vi "Main[Top VI].vi"() -> ()   [LabVIEW 2011]
uses:
  <vilib>/picture/picture.llb/imagedata.ctl
  VIs/sub-Language global.vi
panel:
  out "selected":i32
  out "label4":string="统计数据：通道2"
  out "label3":string="统计数据：通道1"
  out "label2":string="CAN中继状态"
  out "label1":string="CAN发送"
  out "brgsta":u16(ring) caption="CAN中继状态"
  out "Trate2":dbl caption="帧率T:" format="%#.1f"
  out "Rrate2":dbl caption="帧率R:" format="%#.1f"
  out "errcnt2":i32 caption="校验错误:"
  out "Trate1":dbl caption="帧率T:" format="%#.1f"
  in  "path":path
  out "Rrate1":dbl caption="帧率R:" format="%#.1f"
  out "errcnt1":i32 caption="校验错误:"
  in  "reciveEnable":bool=TRUE
  in  "ID Filter Set":bool
  in  "ID Filter Str":string="01 02"
  in  "ID Filter":enum32{"enable", "disable"}(radio)=enum."disable" caption="接收滤波ID设置(直接ID号)"
  in  "savefile":bool
  in  "sendfile":bool
  in  "clear":bool
  in  "send stop":bool
  out "SaveCnt":u32 caption="保存总帧数:"
  in  "Send":bool
  in  "Data Inc":bool
  in  "sendcycle":i32=10 caption="发送周期:" min=0 max=99999999 step=1
  in  "data":string="00 00 00 00 00 00 00 00" caption="数据:"
  in  "ID Inc":bool
  in  "SendCnt":i32=1 caption="发送总帧数:" min=-1
  in  "CAN Channel":u16(ring) caption="CAN通道:" items=["1", "2"]
  in  "Frame ID":string="00 00 00 01" caption="帧ID:"
  in  "Frame Type":u16(ring) caption="帧类型:" items=["数据帧", "远程帧"]
  in  "Frame Format":u16(ring) caption="帧格式:" items=["标准帧", "扩展帧"]
  out "DevIndex":u32
  in  "list":i32(listbox)
  # "ms"
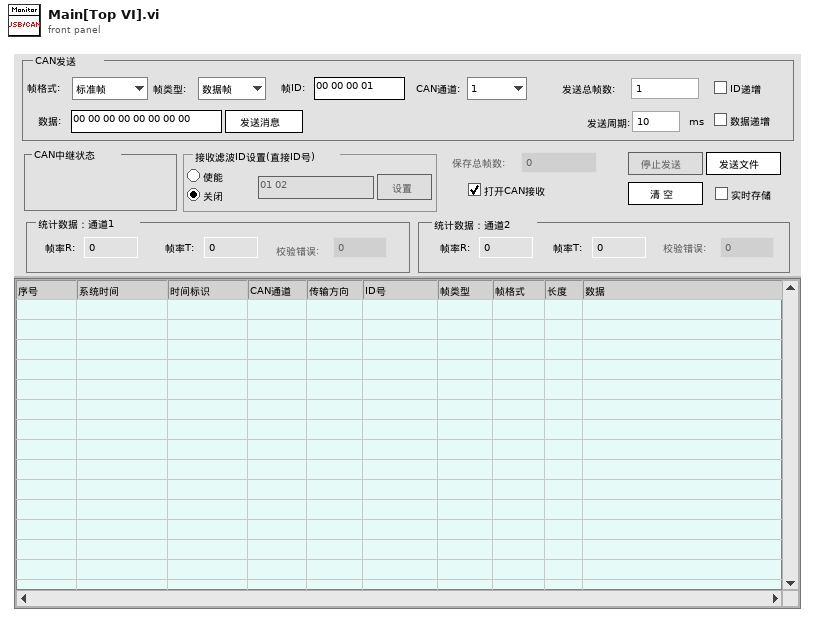
[diagram p1: front panel]
types:
  T1 = enum16{"Init", "RegistEvent", "run", "unRegistEvent", "Release", "Exit"}
  T2 = cluster{"type":u16, "scantime":u16, "highspd":bool, "disp":bool, "save":bool, "hl":bool, "ID合并":bool, "Rfun":u16, "Tfun":u16, "chk1":bool, "chk2":bool, "format":enum16{"hex", "dec", "oct", "bin"}, "rateR1":bool, "rateR2":bool, "rateT1":bool, "rateT2":bool, "RcvE1":bool, "RcvE2":bool, "TSFormat":enum16{"原始值", "实际值"}, "RcvLen":i16, "autoconn":bool, "BuffLen":u16}
  T3 = typedef "imagedata.ctl" = cluster{"image type":i32, "image depth":i32, "image":u8[], "mask":u8[], "colors":u32[], "Rectangle":cluster{"left":i16, "top":i16, "right":i16, "bottom":i16}}
  T4 = enum8{"Enabled", "Disabled", "Disabled and Grayed Out"}
  T5 = typedef "Param.ctl" = cluster{"kCANBAUD":u8, "BTR0":u8, "BTR1":u8, "MODE":u8, "FILTER":u8, "ACR0":u32, "AMR0":u32, "FlashParam":u32, "BAUD":u32, "SJW":u8, "BRP":u8, "SAM":u8, "PHS2_SEL":u8, "PRSEG":u8, "PHSEG1":u8, "PHSEG2":u8}
  T6 = cluster{"desc":string, "appended path":path, "help dir":string}[]
  T7 = cluster{"hw_Version":u16, "fw_Version":u16, "dr_Version":u16, "in_Version":u16, "irq_Num":u16, "can_Num":u8, "str_Serial_Num":string, "str_hw_Type":string, "Reserved":u8[]}
  T8 = cluster{"desc":string, "appended path":path, "help dir":string}
  T9 = enum16{"X", "CAN1--->CAN2", "CAN1<----CAN2", "CAN1<---->CAN2"}
  T10 = typedef "LVPoint32TypeDef.ctl" = cluster{"Horizontal":i32, "Vertical":i32}
  T11 = typedef "LVRowAndColumnTypeDef.ctl" = cluster{"Row":i32, "Column":i32}
  T12 = enum32{"Bad", "Idle", "Run top level", "Running"}
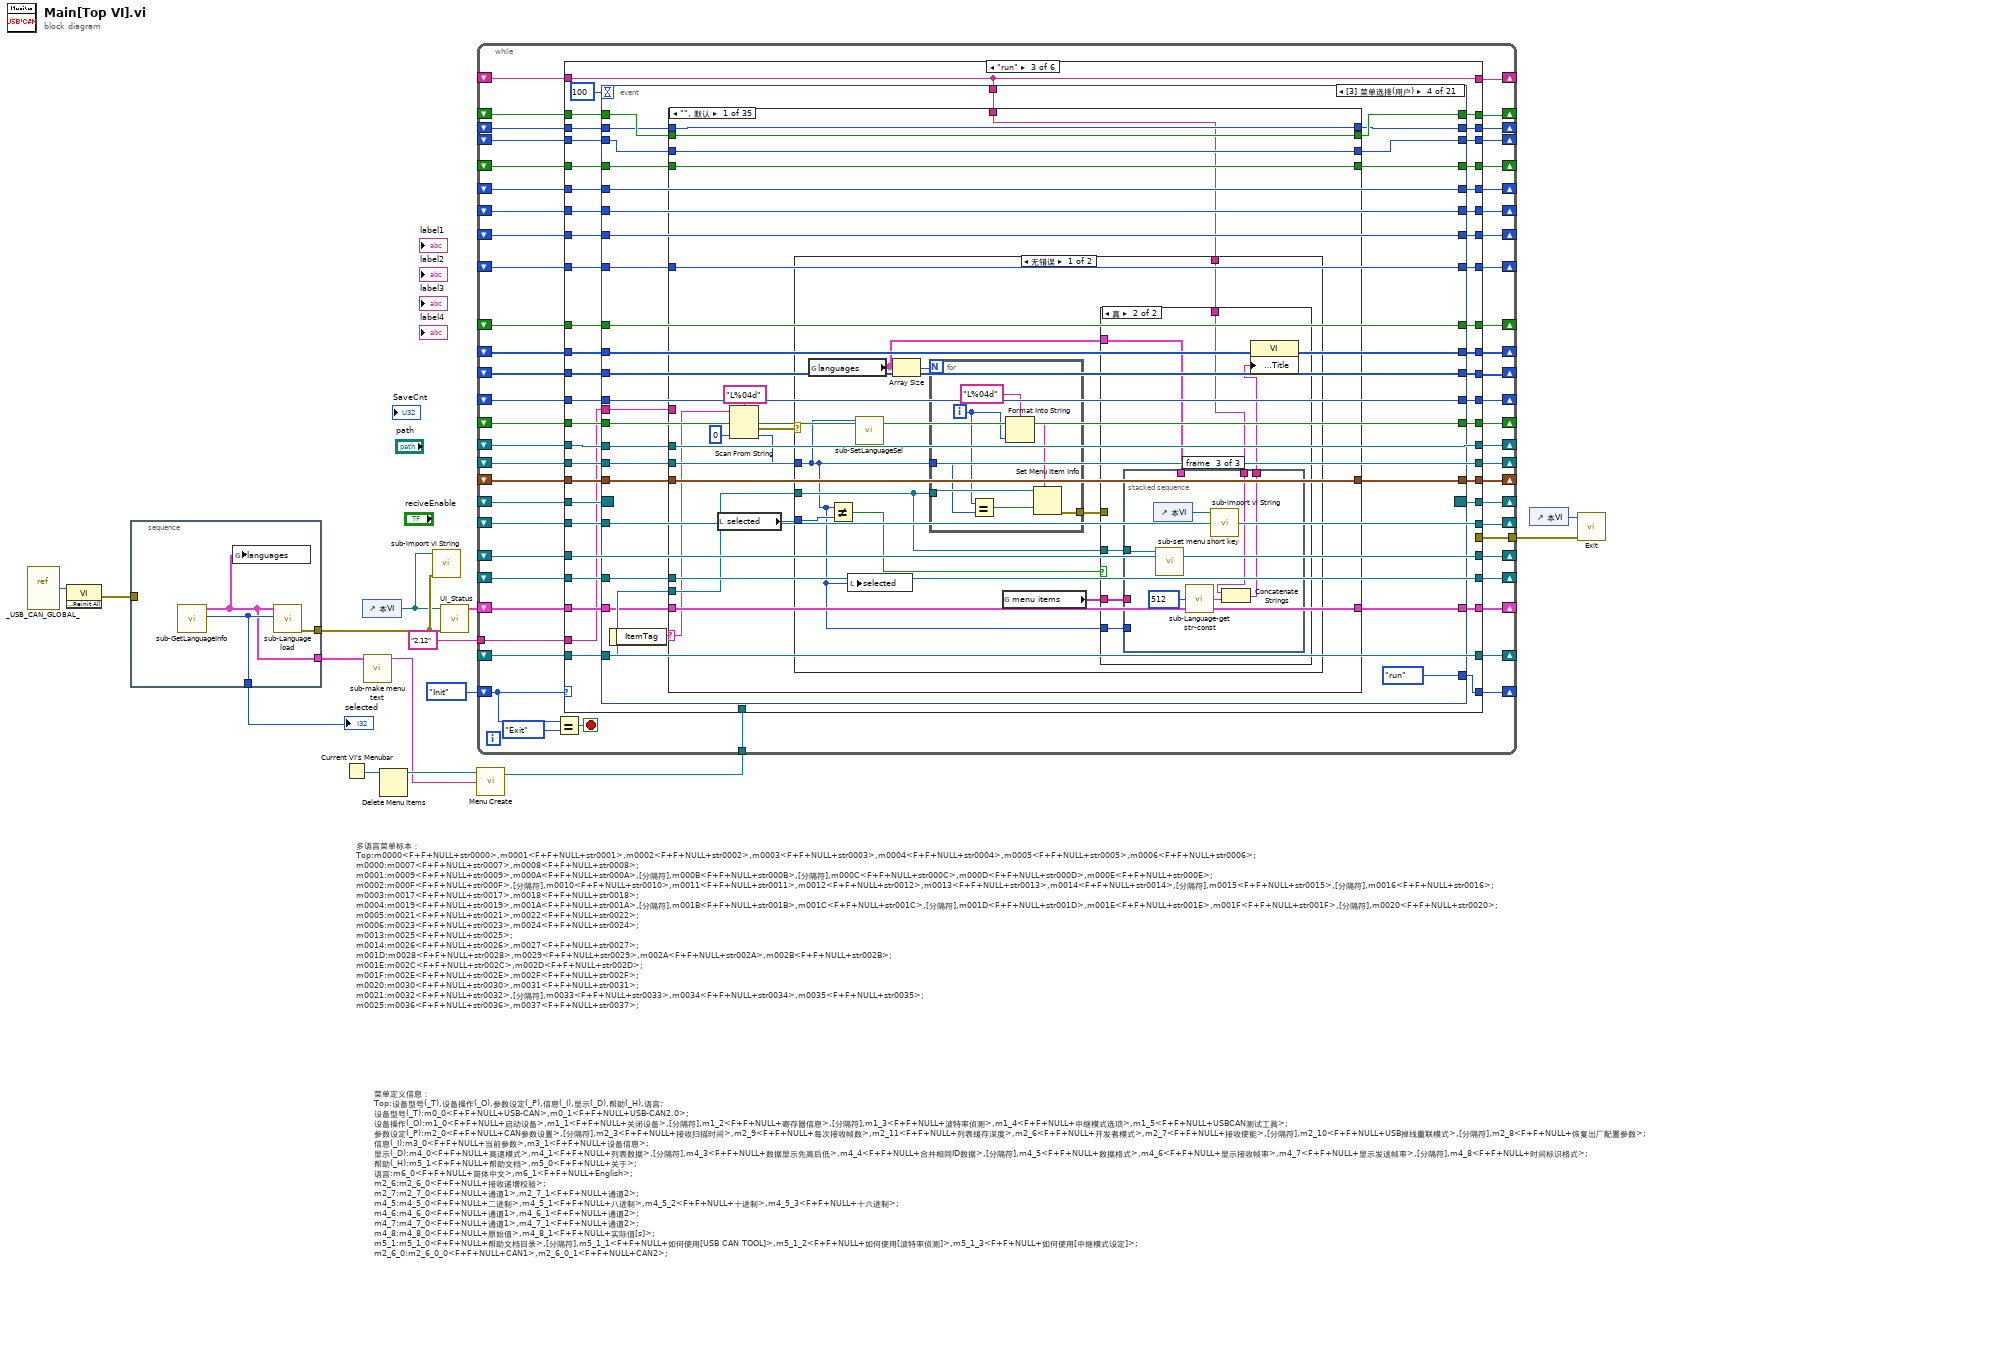
[diagram p0: block diagram]
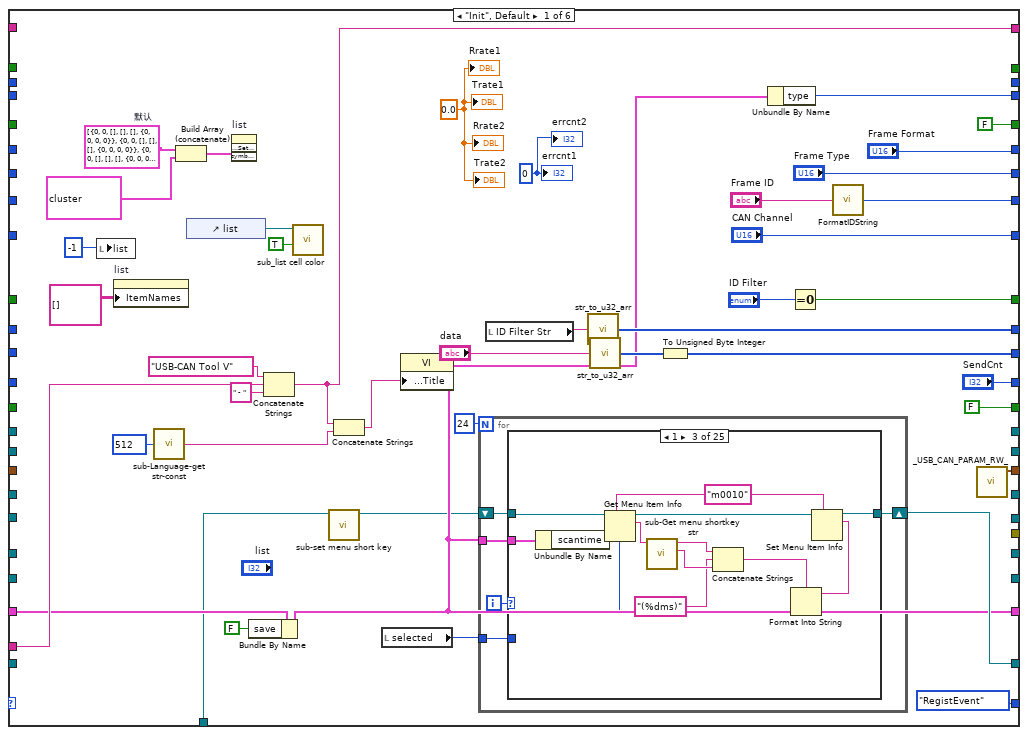
[diagram p2: hidden frame]
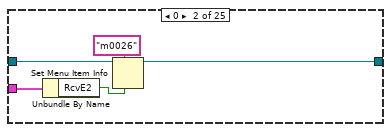
[diagram p4: hidden frame]
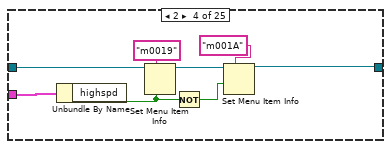
[diagram p5: hidden frame]
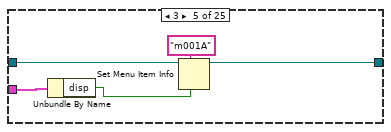
[diagram p6: hidden frame]
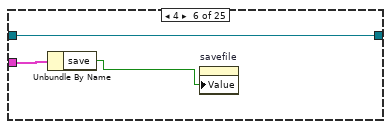
[diagram p7: hidden frame]
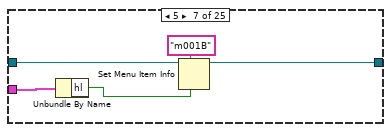
[diagram p8: hidden frame]
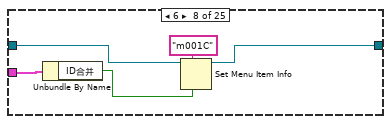
[diagram p9: hidden frame]
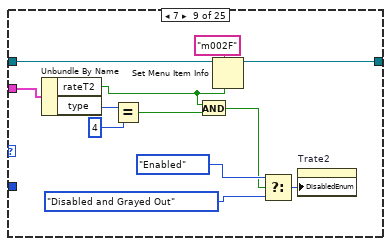
[diagram p10: hidden frame]
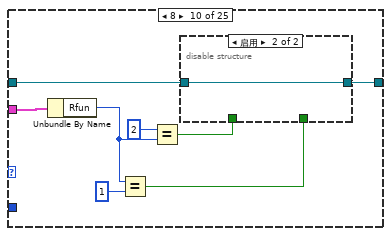
[diagram p11: hidden frame]
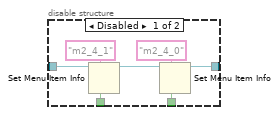
[diagram p12: hidden frame]
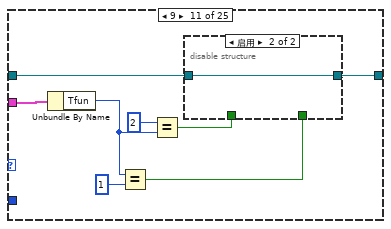
[diagram p13: hidden frame]
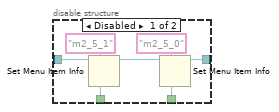
[diagram p14: hidden frame]
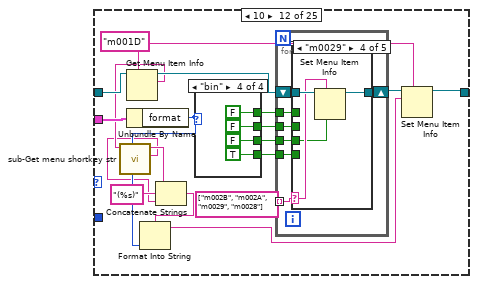
[diagram p15: hidden frame]
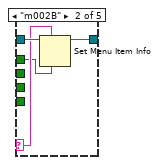
[diagram p17: hidden frame]
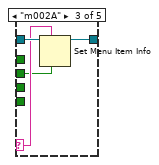
[diagram p18: hidden frame]
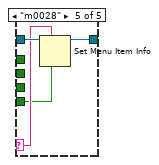
[diagram p19: hidden frame]
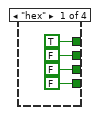
[diagram p20: hidden frame]
diagram:
  # "菜单定义信息：\nTop:设备型号(_T),设备操作(_O),参数设定(_P),信息(_I),显示(_D),帮助(_H),语言;\n设备型号(_T):m0_0<F+F+NULL+USB-CAN>,m0_1<F+F+NULL+USB-CAN2.0>;\n设备操作(_O):m1_0<F+F+NULL+启动设备>,m1_1<F+F+NULL+关闭设备>,[分隔符],m1_2<F+F+NULL+寄存器信息>,[分隔符],m1_3<F+F+NULL+波特率侦测>,m1_4<F+F+NULL+中继模式选项>,m1_5<F+F+NULL+USBCAN测试工具>;\n参数设定(_P):m2_0<F+F+NULL+CAN参数设置>,[分隔符],m2_3<F+F+NULL+接收扫描时间>,m2_9<F+F+NULL+每次接收帧数>,m2_11<F+F+NULL+列表缓存深度>,m2_6<F+F+NULL+开发者模式>,m2_7<F+F+NULL+接收使能>,[分隔符],m2_10<F+F+NULL+USB掉线重联模式>,[分隔符],m2_8<F+F+NULL+恢复出厂配置参数>;\n信息(_I):m3_0<F+F+NULL+当前参数>,m3_1<F+F+NULL+设备信息>;\n显示(_D):m4_0<F+F+NULL+高速模式>,m4_1<F+F+NULL+列表数据>,[分隔符],m4_3<F+F+NULL+数据显示先高后低>,m4_4<F+F+NULL+合并相同ID数据>,[分隔符],m4_5<F+F+NULL+数据格式>,m4_6<F+F+NULL+显示接收帧率>,m4_7<F+F+NULL+显示发送帧率>,[分隔符],m4_8<F+F+NULL+时间标识格式>;\n帮助(_H):m5_1<F+F+NULL+帮助文档>,m5_0<F+F+NULL+关于>;\n语言:m6_0<F+F+NULL+简体中文>,m6_1<F+F+NULL+English>;\nm2_6:m2_6_0<F+F+NULL+接收递增校验>;\nm2_7:m2_7_0<F+F+NULL+通道1>,m2_7_1<F+F+NULL+通道2>;\nm4_5:m4_5_0<F+F+NULL+二进制>,m4_5_1<F+F+NULL+八进制>,m4_5_2<F+F+NULL+十进制>,m4_5_3<F+F+NULL+十六进制>;\nm4_6:m4_6_0<F+F+NULL+通道1>,m4_6_1<F+F+NULL+通道2>;\nm4_7:m4_7_0<F+F+NULL+通道1>,m4_7_1<F+F+NULL+通道2>;\nm4_8:m4_8_0<F+F+NULL+原始值>,m4_8_1<F+F+NULL+实际值[s]>;\nm5_1:m5_1_0<F+F+NULL+帮助文档目录>,[分隔符],m5_1_1<F+F+NULL+如何使用[USB CAN TOOL]>,m5_1_2<F+F+NULL+如何使用[波特率侦测]>,m5_1_3<F+F+NULL+如何使用[中继模式设定]>;\nm2_6_0:m2_6_0_0<F+F+NULL+CAN1>,m2_6_0_1<F+F+NULL+CAN2>;"
  # "多语言菜单标本：\nTop:m0000<F+F+NULL+str0000>,m0001<F+F+NULL+str0001>,m0002<F+F+NULL+str0002>,m0003<F+F+NULL+str0003>,m0004<F+F+NULL+str0004>,m0005<F+F+NULL+str0005>,m0006<F+F+NULL+str0006>;\nm0000:m0007<F+F+NULL+str0007>,m0008<F+F+NULL+str0008>;\nm0001:m0009<F+F+NULL+str0009>,m000A<F+F+NULL+str000A>,[分隔符],m000B<F+F+NULL+str000B>,[分隔符],m000C<F+F+NULL+str000C>,m000D<F+F+NULL+str000D>,m000E<F+F+NULL+str000E>;\nm0002:m000F<F+F+NULL+str000F>,[分隔符],m0010<F+F+NULL+str0010>,m0011<F+F+NULL+str0011>,m0012<F+F+NULL+str0012>,m0013<F+F+NULL+str0013>,m0014<F+F+NULL+str0014>,[分隔符],m0015<F+F+NULL+str0015>,[分隔符],m0016<F+F+NULL+str0016>;\nm0003:m0017<F+F+NULL+str0017>,m0018<F+F+NULL+str0018>;\nm0004:m0019<F+F+NULL+str0019>,m001A<F+F+NULL+str001A>,[分隔符],m001B<F+F+NULL+str001B>,m001C<F+F+NULL+str001C>,[分隔符],m001D<F+F+NULL+str001D>,m001E<F+F+NULL+str001E>,m001F<F+F+NULL+str001F>,[分隔符],m0020<F+F+NULL+str0020>;\nm0005:m0021<F+F+NULL+str0021>,m0022<F+F+NULL+str0022>;\nm0006:m0023<F+F+NULL+str0023>,m0024<F+F+NULL+str0024>;\nm0013:m0025<F+F+NULL+str0025>;\nm0014:m0026<F+F+NULL+str0026>,m0027<F+F+NULL+str0027>;\nm001D:m0028<F+F+NULL+str0028>,m0029<F+F+NULL+str0029>,m002A<F+F+NULL+str002A>,m002B<F+F+NULL+str002B>;\nm001E:m002C<F+F+NULL+str002C>,m002D<F+F+NULL+str002D>;\nm001F:m002E<F+F+NULL+str002E>,m002F<F+F+NULL+str002F>;\nm0020:m0030<F+F+NULL+str0030>,m0031<F+F+NULL+str0031>;\nm0021:m0032<F+F+NULL+str0032>,[分隔符],m0033<F+F+NULL+str0033>,m0034<F+F+NULL+str0034>,m0035<F+F+NULL+str0035>;\nm0025:m0036<F+F+NULL+str0036>,m0037<F+F+NULL+str0037>;"
  n1 = vi-ref "_USB_CAN_GLOBAL_.vi"() -> (w7:refnum<vi>)
  n2 = invoke class="VI" method="Default Vals.Reinit All"(reference=w7) -> (error out=w5:errorcluster)  [unwired: 2 in, 2 out]
  n3 = stacked-sequence {
    tunnel: [w18] -> w10
    tunnel: [w17] -> w8
    tunnel: [w16] -> w6
    tunnel: w5 -> [_]
    frame #0 {
      n4 = call "sub-GetLanguageInfo.vi"() -> ("selected"=w17:i32, "languages"=w16:cluster{string, "appended path":path, string}[])  [unwired: 10 in]
      n5 = global write "sub-Language global.vi" "languages"(w16) -> ()
      n6 = call "sub-Language load.vi"("selected"=w17, "languages"=w16) -> ("error out"=w18:errorcluster)  [unwired: 9 in]
    }
  }
  "selected" <- w8
  n7 = Current VI's Menubar() -> (w4:refnum<k9>)
  n8 = control-ref of="本VI"() -> (w9:refnum<vi>)
  n9 = call "sub-make menu text.vi"("languages"=w6) -> ("menu text"=w2:string)  [unwired: 10 in]
  n10 = Delete Menu Items(9:w4) -> (3:w3:refnum<k9>)  [unwired: 1 in, 3 out]
  n11 = call "sub-import vi String.vi"("error in (no error)"=w10, "vi ref"=w9) -> ()  [unwired: 9 in, 1 out]
  n12 = call "UI_Status.vi"("error in (no error)"=w10, "VI ref"=w9) -> ("menu status in out"=w14:T2)  [unwired: 8 in, 1 out]
  n13 = call "Menu Create.vi"("String"=w2, "menubar in"=w3) -> ("menubar out"=w1:refnum<k9>)  [unwired: 1 in, 1 out]
  n14 = while {
    shift-right: [w68] -> _
    shift-left: T1."Init" -> [w71]
    shift-right: [w67] -> _
    shift-left: _ -> [w66]
    shift-right: [w64] -> _
    shift-left: _ -> [w65]
    shift-right: [w63] -> _
    shift-left: _ -> [w62]
    shift-right: [w61] -> _
    shift-left: _ -> [w60]
    shift-right: [w59] -> _
    shift-left: _ -> [w58]
    shift-right: [w57] -> _
    shift-left: _ -> [w56]
    shift-right: [w55] -> _
    shift-left: _ -> [w54]
    shift-right: [w53] -> _
    shift-left: _ -> [w52]
    shift-right: [w51] -> _
    shift-left: _ -> [w50]
    shift-right: [w49] -> _
    shift-left: _ -> [w48]
    shift-right: [w47] -> _
    shift-left: _ -> [w46]
    shift-right: [w44] -> _
    shift-left: _ -> [w45]
    shift-right: [w43] -> _
    shift-left: _ -> [w42]
    shift-right: [w41] -> _
    shift-left: _ -> [w40]
    shift-right: [w39] -> _
    shift-left: _ -> [w38]
    shift-right: [w37] -> _
    shift-left: _ -> [w35]
    shift-right: [w36] -> _
    shift-left: _ -> [w34]
    tunnel: [w33] -> w13
    shift-right: [w32] -> _
    shift-left: _ -> [w31]
    shift-right: [w30] -> _
    shift-left: w14 -> [w29]
    shift-right: [w28] -> _
    shift-left: _ -> [w27]
    shift-right: [w26] -> _
    shift-left: _ -> [w25]
    shift-right: [w24] -> _
    shift-left: _ -> [w23]
    shift-right: [w22] -> _
    shift-left: _ -> [w21]
    tunnel: "2.12" ("FileVersion") -> [w20]
    tunnel: w1 -> [w19]
    stop <- w69 stop-if-true
    n15 = Equal?(x=w71, y=T1."Exit") -> (x = y?=w69:bool)
    n16 = case shown="\"run\"" w71 {
      tunnel: [T1."RegistEvent" T1."run" w767 T1."Release" T1."Exit" T1."Exit"] -> w68
      tunnel: [FALSE w468 w776 _ _ _] -> w67
      tunnel: w66 -> [_ w468 w785 _ _ _]
      tunnel: w65 -> [_ w467 w784 _ _ _]
      tunnel: ["Frame Format" w467 w775 _ _ _] -> w64
      tunnel: ["Frame Type" w455 w774 _ _ _] -> w63
      tunnel: w62 -> [_ w455 w783 _ _ _]
      tunnel: [w108 w466 w773 _ _ _] -> w61
      tunnel: w60 -> [_ w466 w782 _ _ _]
      tunnel: ["CAN Channel" w454 w772 _ _ _] -> w59
      tunnel: w58 -> [_ w454 w781 _ _ _]
      tunnel: [w84 w441 w770 _ _ _] -> w57
      tunnel: w56 -> [_ w441 w779 _ _ _]
      tunnel: [w105 w442 w771 _ _ _] -> w55
      tunnel: w54 -> [_ w442 w780 _ _ _]
      tunnel: [w99 w465 w769 _ _ _] -> w53
      tunnel: w52 -> [_ w465 w778 _ _ _]
      tunnel: ["SendCnt" w464 w768 _ _ _] -> w51
      tunnel: w50 -> [_ w464 w777 _ _ _]
      tunnel: [FALSE w463 w765 _ _ _] -> w49
      tunnel: w48 -> [_ w463 w766 _ _ _]
      tunnel: [w91 w462 w752 w2340 w2388 _] -> w47
      tunnel: w46 -> [_ w462 w752 w2340 w2388 _]
      tunnel: w45 -> [_ w461 w764 w2334 _ _]
      tunnel: [w86 w461 w763 _ _ _] -> w44
      tunnel: [_ w445 w762 _ _ _] -> w43
      tunnel: w42 -> [_ _ w762 w2358 _ _]
      tunnel: [_ w444 w761 _ _ _] -> w41
      tunnel: w40 -> [_ _ w761 w2351 _ _]
      tunnel: [w96 w456 w759 _ _ _] -> w39
      tunnel: w38 -> [_ w456 w760 w2342 _ _]
      tunnel: [_ w452 w757 _ _ _] -> w37
      tunnel: [_ w451 w756 _ _ _] -> w36
      tunnel: w35 -> [_ _ w758 w2348 _ _]
      tunnel: w34 -> [_ _ w756 w2346 _ _]
      tunnel: [_ _ _ w2345 _ _] -> w33
      tunnel: [_ w446 w755 _ _ _] -> w32
      tunnel: w31 -> [_ _ w755 w2343 _ _]
      tunnel: [w83 w421 w753 w2339 _ _] -> w30
      tunnel: w29 -> [w85 w421 w754 w2339 w2385 _]
      tunnel: [_ FALSE w750 _ _ _] -> w28
      tunnel: w27 -> [_ _ w751 _ _ _]
      tunnel: [_ w433 w749 _ _ _] -> w26
      tunnel: w25 -> [_ _ w749 w2337 _ _]
      tunnel: [_ _ w747 _ _ _] -> w24
      tunnel: w23 -> [_ _ w748 _ _ _]
      tunnel: [w74 w413 w746 w2336 w2384 w2394] -> w22
      tunnel: w21 -> [_ w413 w746 w2336 w2384 w2394]
      tunnel: w20 -> [w89 _ w745 _ _ _]
      tunnel: w19 -> [w77 _ _ _ _ _]
      frame "Init", Default {
        w87 = 0.0 ("rate")
        w95 = T3[] [{"image type"=0, "image depth"=0, "image"=[], "mask"=[], "colors"=[], "Rectangle"={"left"=0, "top"=0, "right"=0, "bottom"=0}}, {"image type"=0, "image depth"=0, "image"=[], "mask"=[], "colors"=[], "Rectangle"={"left"=0, "top"=0, "right"=0, "bottom"=0}}, {"image type"=0, "image depth"=0, "image"=[], "mask"=[], "colors"=[], "Rectangle"={"left"=0, "top"=0, "right"=0, "bottom"=0}}, {"image type"=0, "image depth"=0, "image"=[], "mask"=[], "colors"=[], "Rectangle"={"left"=0, "top"=0, "right"=0, "bottom"=0}}, {"image type"=0, "image depth"=0, "image"=[], "mask"=[], "colors"=[], "Rectangle"={"left"=0, "top"=0, "right"=0, "bottom"=0}}, {"image type"=0, "image depth"=0, "image"=[], "mask"=[], "colors"=[], "Rectangle"={"left"=0, "top"=0, "right"=0, "bottom"=0}}, {"image type"=0, "image depth"=0, "image"=[], "mask"=[], "colors"=[], "Rectangle"={"left"=0, "top"=0, "right"=0, "bottom"=0}}, {"image type"=0, "image depth"=0, "image"=[], "mask"=[], "colors"=[], "Rectangle"={"left"=0, "top"=0, "right"=0, "bottom"=0}}, {"image type"=0, "image depth"=0, "image"=[], "mask"=[], "colors"=[], "Rectangle"={"left"=0, "top"=0, "right"=0, "bottom"=0}}, {"image type"=0, "image depth"=0, "image"=[], "mask"=[], "colors"=[], "Rectangle"={"left"=0, "top"=0, "right"=0, "bottom"=0}}, {"image type"=0, "image depth"=0, "image"=[], "mask"=[], "colors"=[], "Rectangle"={"left"=0, "top"=0, "right"=0, "bottom"=0}}, {"image type"=0, "image depth"=0, "image"=[], "mask"=[], "colors"=[], "Rectangle"={"left"=0, "top"=0, "right"=0, "bottom"=0}}, {"image type"=0, "image depth"=0, "image"=[], "mask"=[], "colors"=[], "Rectangle"={"left"=0, "top"=0, "right"=0, "bottom"=0}}, {"image type"=0, "image depth"=0, "image"=[], "mask"=[], "colors"=[], "Rectangle"={"left"=0, "top"=0, "right"=0, "bottom"=0}}, {"image type"=0, "image depth"=0, "image"=[], "mask"=[], "colors"=[], "Rectangle"={"left"=0, "top"=0, "right"=0, "bottom"=0}}, {"image type"=0, "image depth"=0, "image"=[], "mask"=[], "colors"=[], "Rectangle"={"left"=0, "top"=0, "right"=0, "bottom"=0}}, {"image type"=0, "image depth"=0, "image"=[], "mask"=[], "colors"=[], "Rectangle"={"left"=0, "top"=0, "right"=0, "bottom"=0}}, {"image type"=0, "image depth"=0, "image"=[], "mask"=[], "colors"=[], "Rectangle"={"left"=0, "top"=0, "right"=0, "bottom"=0}}, {"image type"=0, "image depth"=0, "image"=[], "mask"=[], "colors"=[], "Rectangle"={"left"=0, "top"=0, "right"=0, "bottom"=0}}, {"image type"=0, "image depth"=0, "image"=[], "mask"=[], "colors"=[], "Rectangle"={"left"=0, "top"=0, "right"=0, "bottom"=0}}, {"image type"=0, "image depth"=0, "image"=[], "mask"=[], "colors"=[], "Rectangle"={"left"=0, "top"=0, "right"=0, "bottom"=0}}, {"image type"=0, "image depth"=0, "image"=[], "mask"=[], "colors"=[], "Rectangle"={"left"=0, "top"=0, "right"=0, "bottom"=0}}, {"image type"=0, "image depth"=0, "image"=[], "mask"=[], "colors"=[], "Rectangle"={"left"=0, "top"=0, "right"=0, "bottom"=0}}, {"image type"=0, "image depth"=0, "image"=[], "mask"=[], "colors"=[], "Rectangle"={"left"=0, "top"=0, "right"=0, "bottom"=0}}, {"image type"=0, "image depth"=0, "image"=[], "mask"=[], "colors"=[], "Rectangle"={"left"=0, "top"=0, "right"=0, "bottom"=0}}, {"image type"=0, "image depth"=0, "image"=[], "mask"=[], "colors"=[], "Rectangle"={"left"=0, "top"=0, "right"=0, "bottom"=0}}, {"image type"=0, "image depth"=0, "image"=[], "mask"=[], "colors"=[], "Rectangle"={"left"=0, "top"=0, "right"=0, "bottom"=0}}, {"image type"=0, "image depth"=0, "image"=[], "mask"=[], "colors"=[], "Rectangle"={"left"=0, "top"=0, "right"=0, "bottom"=0}}, {"image type"=0, "image depth"=0, "image"=[], "mask"=[], "colors"=[], "Rectangle"={"left"=0, "top"=0, "right"=0, "bottom"=0}}, {"image type"=0, "image depth"=0, "image"=[], "mask"=[], "colors"=[], "Rectangle"={"left"=0, "top"=0, "right"=0, "bottom"=0}}, {"image type"=0, "image depth"=0, "image"=[], "mask"=[], "colors"=[], "Rectangle"={"left"=0, "top"=0, "right"=0, "bottom"=0}}, {"image type"=0, "image depth"=0, "image"=[], "mask"=[], "colors"=[], "Rectangle"={"left"=0, "top"=0, "right"=0, "bottom"=0}}, {"image type"=0, "image depth"=0, "image"=[], "mask"=[], "colors"=[], "Rectangle"={"left"=0, "top"=0, "right"=0, "bottom"=0}}, {"image type"=0, "image depth"=0, "image"=[], "mask"=[], "colors"=[], "Rectangle"={"left"=0, "top"=0, "right"=0, "bottom"=0}}, {"image type"=0, "image depth"=0, "image"=[], "mask"=[], "colors"=[], "Rectangle"={"left"=0, "top"=0, "right"=0, "bottom"=0}}, {"image type"=0, "image depth"=0, "image"=[], "mask"=[], "colors"=[], "Rectangle"={"left"=0, "top"=0, "right"=0, "bottom"=0}}, {"image type"=0, "image depth"=0, "image"=[], "mask"=[], "colors"=[], "Rectangle"={"left"=0, "top"=0, "right"=0, "bottom"=0}}]  # 默认
        w88 = 0 ("errcnt")
        n17 = local write "list"(-1 ("list")) -> ()
        n18 = property on="list" class="MCListbox (严格)"("ItemNames"=string[][] [] ("项名")) -> ()  [unwired: 2 in, 2 out]
        n19 = call "sub-Language-get str-const.vi"("sid"=u32 512) -> ("str"=w73:string)
        n20 = Build Array (concatenate)(w95, T3[] [{"image type"=0, "image depth"=32, "image"=array[1024 elements], "mask"=[255, 255, 255, 255, 255, 255, 255, 255, 255, 255, 255, 255, 255, 255, 255, 255, 255, 255, 255, 255, 255, 255, 255, 255, 255, 255, 255, 255, 255, 255, 255, 255], "colors"=[], "Rectangle"={"left"=0, "top"=0, "right"=16, "bottom"=16}}, {"image type"=0, "image depth"=32, "image"=array[1024 elements], "mask"=[255, 255, 255, 255, 255, 255, 255, 255, 255, 255, 255, 255, 255, 255, 255, 255, 255, 255, 255, 255, 255, 255, 255, 255, 255, 255, 255, 255, 255, 255, 255, 255], "colors"=[], "Rectangle"={"left"=0, "top"=0, "right"=16, "bottom"=16}}] ("数组")) -> (w94:T3[])
        n21 = control-ref of="list"() -> (w81:refnum<vi>)
        n22 = invoke on="list" class="MCListbox (严格)" method="Custom Item Symbols.Set Symbol Array"("symbols"=w94) -> ()  [unwired: 3 in, 4 out]
        n23 = Bundle By Name(cluster=w85, "save"=FALSE) -> (w83:T2)
        n24 = Concatenate Strings("USB-CAN Tool V", w89, " - " ("字符串")) -> (w74:string)
        n25 = call "sub_list cell color.vi"("Reset?(F)"=TRUE, "list ref"=w81) -> ()  [unwired: 8 in, 2 out]
        n26 = call "sub-set menu short key.vi"("menubar in"=w77) -> ("menubar out"=w78:refnum<k9>)  [unwired: 9 in, 1 out]
        n27 = Concatenate Strings(w74, w73) -> (w72:string)
        n28 = local read "selected"() -> (w79:i32)
        n29 = property class="VI"("Front Panel.Title"=w72) -> ()  [unwired: 2 in, 2 out]
        n30 = for {
          N: 24 -> [_]
          shift-right: [w115] -> w91
          shift-left: w78 -> [w116]
          tunnel: w83 -> [w117]
          tunnel: w79 -> [w114]
          i -> [w118]
          n31 = case shown="1" w118 {
            tunnel: w117 -> [_ w124 w136 w144 w149 w152 w157 w162 w174 w182 w198 w224 w272 w284 w292 w304 w312 w317 w334 _ w370 w387 w399 w402 _]
            tunnel: w116 -> [w119 w123 w132 w143 w148 w151 w156 w161 w173 w181 w197 w214 w271 w283 w291 w303 w311 w316 w332 w357 w376 w384 w396 w405 w411]
            tunnel: [w119 w121 w135 w140 w147 w151 w155 w160 w171 w180 w196 w217 w269 w281 w289 w301 w309 w314 w331 w356 w372 w388 w400 w404 w410] -> w115
            tunnel: w114 -> [_ _ _ _ _ _ _ _ _ _ _ _ _ _ _ _ _ _ _ _ _ _ _ _ w409]
            frame -1, Default {
            }
            frame 0 {
              n32 = Unbundle By Name(w124) -> ("RcvE2"=w120:bool)
              n33 = Set Menu Item Info(6:w120, 7:"m0026" ("项标识符"), 11:w123) -> (3:w121:refnum<k9>)  [unwired: 4 in, 1 out]
            }
            frame 1 {
              w130 = "m0010" ("项标识符")
              n34 = Unbundle By Name(w136) -> ("scantime"=w134:u16)
              n35 = Get Menu Item Info(7:w130, 11:w132) -> (2:w129:string, 3:w131:refnum<k9>)  [unwired: 1 in, 5 out]
              n36 = call "sub-Get menu shortkey str.vi"("menu desc"=w129) -> ("short key str"=w127:string, "menu desc split"=w128:string)  [unwired: 9 in]
              n37 = Concatenate Strings(w128, "(%dms)" ("格式字符串"), w127) -> (w125:string)
              n38 = Format Into String(format string=w125, w134) -> (resulting string=w133:string)  [unwired: 2 in, 1 out]
              n39 = Set Menu Item Info(7:w130, 10:w133, 11:w131) -> (3:w135:refnum<k9>)  [unwired: 4 in, 1 out]
            }
            frame 2 {
              n40 = Unbundle By Name(w144) -> ("highspd"=w138:bool)
              n41 = Set Menu Item Info(6:w138, 7:"m0019" ("项标识符"), 11:w143) -> (3:w141:refnum<k9>)  [unwired: 4 in, 1 out]
              n42 = Not(x=w138) -> (.not. x?=w137:bool)
              n43 = Set Menu Item Info(7:"m001A" ("项标识符"), 9:w137, 11:w141) -> (3:w140:refnum<k9>)  [unwired: 4 in, 1 out]
            }
            frame 3 {
              n44 = Unbundle By Name(w149) -> ("disp"=w145:bool)
              n45 = Set Menu Item Info(6:w145, 7:"m001A" ("项标识符"), 11:w148) -> (3:w147:refnum<k9>)  [unwired: 4 in, 1 out]
            }
            frame 4 {
              n46 = Unbundle By Name(w152) -> ("save"=w150:bool)
              n47 = property on="savefile" class="Bool (严格)"("Value"=w150) -> ()  [unwired: 2 in, 2 out]
            }
            frame 5 {
              n48 = Unbundle By Name(w157) -> ("hl"=w153:bool)
              n49 = Set Menu Item Info(6:w153, 7:"m001B" ("项标识符"), 11:w156) -> (3:w155:refnum<k9>)  [unwired: 4 in, 1 out]
            }
            frame 6 {
              n50 = Unbundle By Name(w162) -> ("ID合并"=w158:bool)
              n51 = Set Menu Item Info(6:w158, 7:"m001C" ("项标识符"), 11:w161) -> (3:w160:refnum<k9>)  [unwired: 4 in, 1 out]
            }
            frame 7 {
              n52 = Unbundle By Name(w174) -> ("rateT2"=w165:bool, "type"=w167:u16)
              n53 = Equal?(x=w167, y=u16 4) -> (x = y?=w164:bool)
              n54 = And(x=w165, y=w164) -> (x .and. y?=w163:bool)
              n55 = Set Menu Item Info(6:w165, 7:"m002F" ("项标识符"), 11:w173) -> (3:w171:refnum<k9>)  [unwired: 4 in, 1 out]
              n56 = Select(t=T4."Enabled" ("禁用"), s=w163, f=T4."Disabled and Grayed Out" ("禁用")) -> (s? t:f=w169:T4)
              n57 = property on="Trate2" class="DigNum (严格)"("DisabledEnum"=w169) -> ()  [unwired: 2 in, 2 out]
            }
            frame 8 {
              n58 = Unbundle By Name(w182) -> ("Rfun"=w177:u16)
              n59 = Equal?(x=w177, y=u16 1) -> (x = y?=w178:bool)
              n60 = Equal?(x=u16 2, y=w177) -> (x = y?=w175:bool)
              n61 = disable-structure shown="启用" {
                disable-tunnel: w181 -> [w189 w190]
                disable-tunnel: [w185 w190] -> w180
                disable-tunnel: w178 -> [w184 _]
                disable-tunnel: w175 -> [w183 _]
                frame Disabled {
                  n62 = Set Menu Item Info(6:w183, 7:"m2_4_1" ("项标识符"), 11:w189) -> (3:w186:refnum<k9>)  [unwired: 4 in, 1 out]
                  n63 = Set Menu Item Info(6:w184, 7:"m2_4_0" ("项标识符"), 11:w186) -> (3:w185:refnum<k9>)  [unwired: 4 in, 1 out]
                }
                frame Enabled {
                }
              }
            }
            frame 9 {
              n64 = Unbundle By Name(w198) -> ("Tfun"=w193:u16)
              n65 = Equal?(x=w193, y=u16 1) -> (x = y?=w194:bool)
              n66 = Equal?(x=u16 2, y=w193) -> (x = y?=w191:bool)
              n67 = disable-structure shown="启用" {
                disable-tunnel: w197 -> [w205 w206]
                disable-tunnel: [w201 w206] -> w196
                disable-tunnel: w194 -> [w200 _]
                disable-tunnel: w191 -> [w199 _]
                frame Disabled {
                  n68 = Set Menu Item Info(6:w199, 7:"m2_5_1" ("项标识符"), 11:w205) -> (3:w202:refnum<k9>)  [unwired: 4 in, 1 out]
                  n69 = Set Menu Item Info(6:w200, 7:"m2_5_0" ("项标识符"), 11:w202) -> (3:w201:refnum<k9>)  [unwired: 4 in, 1 out]
                }
                frame Enabled {
                }
              }
            }
            frame 10 {
              w212 = "m001D" ("项标识符")
              n70 = Get Menu Item Info(7:w212, 11:w214) -> (2:w211:string, 3:w213:refnum<k9>)  [unwired: 1 in, 5 out]
              n71 = call "sub-Get menu shortkey str.vi"("menu desc"=w211) -> ("short key str"=w208:string, "menu desc split"=w210:string)  [unwired: 9 in]
              n72 = Unbundle By Name(w224) -> ("format"=w219:enum16{"hex", "dec", "oct", "bin"})
              n73 = Concatenate Strings(w210, "(%s)" ("字符串"), w208) -> (w207:string)
              n74 = Format Into String(format string=w207, w219) -> (resulting string=w216:string)  [unwired: 2 in, 1 out]
              n75 = case shown="\"bin\"" w219 {
                tunnel: [TRUE FALSE FALSE FALSE] -> w223
                tunnel: [FALSE TRUE FALSE FALSE] -> w222
                tunnel: [FALSE FALSE TRUE FALSE] -> w221
                tunnel: [FALSE FALSE FALSE TRUE] -> w220
                frame "hex" {
                }
                frame "dec" {
                }
                frame "oct" {
                }
                frame "bin" {
                }
              }
              n76 = for {
                shift-right: [w230] -> w218
                shift-left: w213 -> [w231]
                tunnel: string[] ["m002B", "m002A", "m0029", "m0028"] -> [w229] mode=indexing
                tunnel: w223 -> [w228]
                tunnel: w222 -> [w227]
                tunnel: w221 -> [w226]
                tunnel: w220 -> [w225]
                n77 = case shown="\"m0029\"" w229 {
                  selector: w229 -> [_ w234 w238 w242 w246]
                  tunnel: w231 -> [w232 w236 w240 w244 w248]
                  tunnel: [w232 w235 w239 w243 w247] -> w230
                  tunnel: w228 -> [_ w233 _ _ _]
                  tunnel: w227 -> [_ _ w237 _ _]
                  tunnel: w226 -> [_ _ _ w241 _]
                  tunnel: w225 -> [_ _ _ _ w245]
                  frame "", Default {
                  }
                  frame "m002B" {
                    n78 = Set Menu Item Info(6:w233, 7:w234, 11:w236) -> (3:w235:refnum<k9>)  [unwired: 4 in, 1 out]
                  }
                  frame "m002A" {
                    n79 = Set Menu Item Info(6:w237, 7:w238, 11:w240) -> (3:w239:refnum<k9>)  [unwired: 4 in, 1 out]
                  }
                  frame "m0029" {
                    n80 = Set Menu Item Info(6:w241, 7:w242, 11:w244) -> (3:w243:refnum<k9>)  [unwired: 4 in, 1 out]
                  }
                  frame "m0028" {
                    n81 = Set Menu Item Info(6:w245, 7:w246, 11:w248) -> (3:w247:refnum<k9>)  [unwired: 4 in, 1 out]
                  }
                }
              }
              n82 = Set Menu Item Info(7:w212, 10:w216, 11:w218) -> (3:w217:refnum<k9>)  [unwired: 4 in, 1 out]
            }
            frame 11 {
              n83 = Unbundle By Name(w272) -> ("chk1"=w265:bool)
              n84 = Set Menu Item Info(6:w265, 7:"m0036" ("项标识符"), 11:w271) -> (3:w269:refnum<k9>)  [unwired: 4 in, 1 out]
              n85 = Select(t=T4."Enabled" ("禁用"), s=w265, f=T4."Disabled and Grayed Out" ("禁用")) -> (s? t:f=w267:T4)
              n86 = property on="errcnt1" class="DigNum (严格)"("DisabledEnum"=w267) -> ()  [unwired: 2 in, 2 out]
            }
            frame 12 {
              n87 = Unbundle By Name(w284) -> ("chk2"=w275:bool, "type"=w277:u16)
              n88 = Equal?(x=w277, y=u16 4) -> (x = y?=w274:bool)
              n89 = And(x=w275, y=w274) -> (x .and. y?=w273:bool)
              n90 = Set Menu Item Info(6:w275, 7:"m0037" ("项标识符"), 11:w283) -> (3:w281:refnum<k9>)  [unwired: 4 in, 1 out]
              n91 = Select(t=T4."Enabled" ("禁用"), s=w273, f=T4."Disabled and Grayed Out" ("禁用")) -> (s? t:f=w279:T4)
              n92 = property on="errcnt2" class="DigNum (严格)"("DisabledEnum"=w279) -> ()  [unwired: 2 in, 2 out]
            }
            frame 13 {
              n93 = Unbundle By Name(w292) -> ("rateR1"=w285:bool)
              n94 = Set Menu Item Info(6:w285, 7:"m002C" ("项标识符"), 11:w291) -> (3:w289:refnum<k9>)  [unwired: 4 in, 1 out]
              n95 = Select(t=T4."Enabled" ("禁用"), s=w285, f=T4."Disabled and Grayed Out" ("禁用")) -> (s? t:f=w287:T4)
              n96 = property on="Rrate1" class="DigNum (严格)"("DisabledEnum"=w287) -> ()  [unwired: 2 in, 2 out]
            }
            frame 14 {
              n97 = Unbundle By Name(w304) -> ("rateR2"=w295:bool, "type"=w297:u16)
              n98 = Equal?(x=w297, y=u16 4) -> (x = y?=w294:bool)
              n99 = And(x=w295, y=w294) -> (x .and. y?=w293:bool)
              n100 = Set Menu Item Info(6:w295, 7:"m002D" ("项标识符"), 11:w303) -> (3:w301:refnum<k9>)  [unwired: 4 in, 1 out]
              n101 = Select(t=T4."Enabled" ("禁用"), s=w293, f=T4."Disabled and Grayed Out" ("禁用")) -> (s? t:f=w299:T4)
              n102 = property on="Rrate2" class="DigNum (严格)"("DisabledEnum"=w299) -> ()  [unwired: 2 in, 2 out]
            }
            frame 15 {
              n103 = Unbundle By Name(w312) -> ("rateT1"=w306:bool)
              n104 = Set Menu Item Info(6:w306, 7:"m002E" ("项标识符"), 11:w311) -> (3:w309:refnum<k9>)  [unwired: 4 in, 1 out]
              n105 = Select(t=T4."Enabled" ("禁用"), s=w306, f=T4."Disabled and Grayed Out" ("禁用")) -> (s? t:f=w307:T4)
              n106 = property on="Trate1" class="DigNum (严格)"("DisabledEnum"=w307) -> ()  [unwired: 2 in, 2 out]
            }
            frame 16 {
              n107 = Unbundle By Name(w317) -> ("RcvE1"=w313:bool)
              n108 = Set Menu Item Info(6:w313, 7:"m0026" ("项标识符"), 11:w316) -> (3:w314:refnum<k9>)  [unwired: 4 in, 1 out]
            }
            frame 17 {
              n109 = Unbundle By Name(w334) -> ("type"=w333:u16, "rateR2"=w321:bool, "rateT2"=w320:bool, "chk2"=w319:bool)
              n110 = case shown="默认" w333 {
                tunnel: w332 -> [w337 w343 w355]
                tunnel: [w337 w340 w353] -> w327
                tunnel: [_ _ w352] -> w326
                tunnel: [w336 w339 w351] -> w323
                tunnel: [w336 w339 w349] -> w324
                tunnel: [w336 w339 w347] -> w322
                tunnel: w321 -> [_ _ w350]
                tunnel: w320 -> [_ _ w348]
                tunnel: w319 -> [_ _ w346]
                tunnel: [i32[] [1] ("禁用项[]") i32[] [1] ("禁用项[]") _] -> w318
                frame Default {
                  w336 = 2
                }
                frame 3 {
                  w339 = 2
                  n111 = Set Menu Item Info(6:TRUE ("已勾选"), 7:"m0007" ("项标识符"), 11:w343) -> (3:w340:refnum<k9>)  [unwired: 4 in, 1 out]
                }
                frame 4 {
                  w344 = 2
                  w345 = 0
                  w352 = TRUE ("已勾选")
                  n112 = Set Menu Item Info(6:w352, 7:"m0008" ("项标识符"), 11:w355) -> (3:w353:refnum<k9>)  [unwired: 4 in, 1 out]
                  n113 = Select(t=w345, s=w348, f=w344) -> (s? t:f=w349:i32)
                  n114 = Select(t=w345, s=w350, f=w344) -> (s? t:f=w351:i32)
                  n115 = Select(t=w345, s=w346, f=w344) -> (s? t:f=w347:i32)
                }
              }
              n116 = property on="CAN Channel" class="Ring (严格)"("Disabled Items []"=w318) -> ()  [unwired: 2 in, 2 out]
              n117 = property on="Trate2" class="DigNum (严格)"("DisabledEnum"=w324) -> ()  [unwired: 2 in, 2 out]
              n118 = property on="Rrate2" class="DigNum (严格)"("DisabledEnum"=w323) -> ()  [unwired: 2 in, 2 out]
              n119 = property on="errcnt2" class="DigNum (严格)"("DisabledEnum"=w322) -> ()  [unwired: 2 in, 2 out]
              n120 = Set Menu Item Info(7:"m0037" ("项标识符"), 9:w326, 11:w327) -> (3:w331:refnum<k9>)  [unwired: 4 in, 1 out]
              n121 = Set Menu Item Info(7:"m0027" ("项标识符"), 9:w326, 11:w327) -> ()  [unwired: 4 in, 2 out]
              n122 = Set Menu Item Info(7:"m002D" ("项标识符"), 9:w326, 11:w327) -> ()  [unwired: 4 in, 2 out]
              n123 = Set Menu Item Info(7:"m002F" ("项标识符"), 9:w326, 11:w327) -> ()  [unwired: 4 in, 2 out]
            }
            frame 18 {
              n124 = disable-structure shown="启用" {
                disable-tunnel: w357 -> [w364 w365]
                disable-tunnel: [w360 w365] -> w356
                frame Disabled {
                  w358 = FALSE ("已启用")
                  n125 = Set Menu Item Info(7:"m2_4" ("项标识符"), 9:w358, 11:w364) -> (0:w361:errorcluster, 3:w362:refnum<k9>)  [unwired: 4 in]
                  n126 = Set Menu Item Info(7:"m2_5" ("项标识符"), 8:w361, 9:w358, 11:w362) -> (3:w360:refnum<k9>)  [unwired: 3 in, 1 out]
                }
                frame Enabled {
                }
              }
            }
            frame 19 {
              n127 = Unbundle By Name(w370) -> ("TSFormat"=w369:enum16{"原始值", "实际值"})
              n128 = Equal?(x=w369, y=enum16{"原始值", "实际值"}."原始值") -> (x = y?=w367:bool)
              n129 = Set Menu Item Info(6:w367, 7:"m0030" ("项标识符"), 11:w376) -> (0:w373:errorcluster, 3:w374:refnum<k9>)  [unwired: 4 in]
              n130 = Not(x=w367) -> (.not. x?=w366:bool)
              n131 = Set Menu Item Info(6:w366, 7:"m0031" ("项标识符"), 8:w373, 11:w374) -> (3:w372:refnum<k9>)  [unwired: 3 in, 1 out]
            }
            frame 20 {
              w382 = "m0011" ("项标识符")
              n132 = Unbundle By Name(w387) -> ("RcvLen"=w386:i16)
              n133 = Get Menu Item Info(7:w382, 11:w384) -> (2:w381:string, 3:w383:refnum<k9>)  [unwired: 1 in, 5 out]
              n134 = call "sub-Get menu shortkey str.vi"("menu desc"=w381) -> ("short key str"=w379:string, "menu desc split"=w380:string)  [unwired: 9 in]
              n135 = Concatenate Strings(w380, "(%d)" ("格式字符串"), w379) -> (w377:string)
              n136 = Format Into String(format string=w377, w386) -> (resulting string=w385:string)  [unwired: 2 in, 1 out]
              n137 = Set Menu Item Info(7:w382, 10:w385, 11:w383) -> (3:w388:refnum<k9>)  [unwired: 4 in, 1 out]
            }
            frame 22 {
              w394 = "m0012" ("项标识符")
              n138 = Unbundle By Name(w399) -> ("BuffLen"=w398:u16)
              n139 = Get Menu Item Info(7:w394, 11:w396) -> (2:w393:string, 3:w395:refnum<k9>)  [unwired: 1 in, 5 out]
              n140 = call "sub-Get menu shortkey str.vi"("menu desc"=w393) -> ("short key str"=w391:string, "menu desc split"=w392:string)  [unwired: 9 in]
              n141 = Concatenate Strings(w392, "(%d)" ("格式字符串"), w391) -> (w389:string)
              n142 = Format Into String(format string=w389, w398) -> (resulting string=w397:string)  [unwired: 2 in, 1 out]
              n143 = Set Menu Item Info(7:w394, 10:w397, 11:w395) -> (3:w400:refnum<k9>)  [unwired: 4 in, 1 out]
            }
            frame 21 {
              n144 = Unbundle By Name(w402) -> ("autoconn"=w401:bool)
              n145 = Set Menu Item Info(6:w401, 7:"m0015" ("项标识符"), 11:w405) -> (3:w404:refnum<k9>)  [unwired: 4 in, 1 out]
            }
            frame 23 {
              n146 = Format Into String(format string="L%04d" ("格式字符串"), w409) -> (resulting string=w407:string)  [unwired: 2 in, 1 out]
              n147 = Set Menu Item Info(6:TRUE ("已勾选"), 7:w407, 11:w411) -> (3:w410:refnum<k9>)  [unwired: 4 in, 1 out]
            }
          }
        }
        n148 = local read "ID Filter Str"() -> (w98:string)
        n149 = call "str_to_u32_arr.vi"("string"=w98) -> ("array"=w84:u32[])
        n150 = call "str_to_u32_arr.vi"("string"="data") -> ("array"=w100:u32[])
        n151 = To Unsigned Byte Integer(number=w100) -> (unsigned 8bit integer=w99:u8[])
        n152 = Unbundle By Name(w83) -> ("type"=w86:u16)
        n153 = Equal To 0?(x="ID Filter") -> (x = 0?=w105:bool)
        n154 = call "FormatIDString.vi"("ID String"="Frame ID") -> ("ID"=w108:u32)
        n155 = call "_USB_CAN_PARAM_RW_.vi"() -> ("param out"=w96:T5[])  [unwired: 11 in]
        "errcnt1" <- w88
        "Rrate1" <- w87
        "Trate1" <- w87
        "errcnt2" <- w88
        "Rrate2" <- w87
        "Trate2" <- w87
      }
      frame "RegistEvent" {
        w434 = TRUE  # openCan
        w450 = TRUE  # savecancel
        w453 = TRUE  # sendover
        n156 = local read "reciveEnable"() -> (w431:bool)
        n157 = Unbundle By Name(w421) -> ("Rfun"=w437:u16, "Tfun"=w432:u16, "hl"=w430:bool, "scantime"=w426:u16)
        n158 = Open VI Reference(vi path=path "DeviceOP/ReciveThread.vi" ("VI路径")) -> (vi reference=w439:refnum<vi>, error out=w436:errorcluster)  [unwired: 5 in]
        n159 = global write "_USB_CAN_GLOBAL_.vi" "R-Enb"(w431) -> ()
        n160 = local write "brgsta"(u16 0 ("brgsta")) -> ()
        n161 = invoke class="VI" method="Ctrl Val.Set"(reference=w439, error in=w436, "Control Name"="RFun" ("控件名"), "Value"=w437) -> (reference out=w429:refnum<vi>, error out=w428:errorcluster)  [unwired: 1 in, 3 out]
        n162 = global write "_USB_CAN_GLOBAL_.vi" "Disp-HL"(w430) -> ()
        n163 = Open VI Reference(vi path=path "VIs/UpdateCANData.vi" ("VI路径"), options=0 ("选项")) -> (vi reference=w449:refnum<vi>, error out=w448:errorcluster)  [unwired: 4 in]
        n164 = Open VI Reference(vi path=path "VIs/CAN_DEBUG_Send.vi" ("VI路径")) -> (vi reference=w458:refnum<vi>, error out=w457:errorcluster)  [unwired: 5 in]
        n165 = invoke class="VI" method="Ctrl Val.Set"(reference=w429, error in=w428, "Control Name"="Scan time" ("控件名"), "Value"=w426) -> (reference out=w423:refnum<vi>, error out=w422:errorcluster)  [unwired: 1 in, 3 out]
        n166 = Create User Event(user event datatype=w450) -> (user event=w446:refnum<user-event>)  [unwired: 1 in, 1 out]
        n167 = for {
          N: 28 -> [_]
          shift-right: [w561] -> w445
          shift-left: w449 -> [w563]
          shift-right: [w560] -> w418
          shift-left: w448 -> [w562]
          tunnel: w446 -> [w559]
          tunnel: w421 -> [w558]
          tunnel: w442 -> [w557]
          tunnel: w441 -> [w556]
          i -> [w564]
          n168 = case shown="-1, 默认" w564 {
            tunnel: w563 -> [w566 w570 w576 w581 w588 w594 w600 w606 w613 w620 w627 w634 w640 w646 w652 w658 w665 w670 w677 w683 w689 w696 w703 w710 w717 w724 w731 w738 w743]
            tunnel: w562 -> [w565 w569 w575 w579 w586 w593 w599 w605 w612 w619 w626 w633 w639 w645 w651 w657 w664 w668 w676 w682 w688 w695 w702 w709 w716 w723 w730 w737 w742]
            tunnel: [w566 w567 w574 w578 w587 w592 w598 w604 w611 w618 w625 w632 w638 w644 w650 w656 w663 w667 w675 w681 w687 w694 w701 w708 w715 w722 w729 w736 w741] -> w561
            tunnel: [w565 w568 w573 w577 w585 w591 w597 w603 w610 w617 w624 w631 w637 w643 w649 w655 w662 w666 w674 w680 w686 w693 w700 w707 w714 w721 w728 w735 w740] -> w560
            tunnel: w559 -> [_ _ _ _ _ _ w595 _ _ _ _ _ _ _ _ _ _ _ _ _ _ _ _ _ _ _ _ _ _]
            tunnel: w558 -> [_ _ _ _ _ _ _ _ w608 w615 w622 w629 _ _ _ _ w660 _ _ _ _ w691 w698 w705 w712 w719 w726 w733 _]
            tunnel: w557 -> [_ _ _ _ _ _ _ _ _ _ _ _ _ _ w647 _ _ _ _ _ _ _ _ _ _ _ _ _ _]
            tunnel: w556 -> [_ _ _ _ _ _ _ _ _ _ _ _ _ _ _ w653 _ _ _ _ _ _ _ _ _ _ _ _ _]
            frame -1, Default {
            }
            frame 0 {
              n169 = invoke class="VI" method="Default Vals.Reinit All"(reference=w570, error in=w569) -> (reference out=w567:refnum<vi>, error out=w568:errorcluster)  [unwired: 1 in, 1 out]
            }
            frame 1 {
              n170 = control-ref of="list"() -> (w571:refnum<vi>)
              n171 = invoke class="VI" method="Ctrl Val.Set"(reference=w576, error in=w575, "Control Name"="list ref" ("控件名"), "Value"=w571) -> (reference out=w574:refnum<vi>, error out=w573:errorcluster)  [unwired: 1 in, 3 out]
            }
            frame 2 {
              n172 = control-ref of="errcnt1"() -> (w580:refnum<vi>)
              n173 = invoke class="VI" method="Ctrl Val.Set"(reference=w581, error in=w579, "Control Name"="errcnt1" ("控件名"), "Value"=w580) -> (reference out=w578:refnum<vi>, error out=w577:errorcluster)  [unwired: 1 in, 3 out]
            }
            frame 3 {
              n174 = control-ref of="本VI"() -> (w583:refnum<vi>)
              n175 = invoke class="VI" method="Ctrl Val.Set"(reference=w588, error in=w586, "Control Name"="vi ref" ("控件名"), "Value"=w583) -> (reference out=w587:refnum<vi>, error out=w585:errorcluster)  [unwired: 1 in, 3 out]
            }
            frame 4 {
              n176 = control-ref of="Rrate1"() -> (w589:refnum<vi>)
              n177 = invoke class="VI" method="Ctrl Val.Set"(reference=w594, error in=w593, "Control Name"="rate0" ("控件名"), "Value"=w589) -> (reference out=w592:refnum<vi>, error out=w591:errorcluster)  [unwired: 1 in, 3 out]
            }
            frame 5 {
              n178 = invoke class="VI" method="Ctrl Val.Set"(reference=w600, error in=w599, "Control Name"="cancelEvt" ("控件名"), "Value"=w595) -> (reference out=w598:refnum<vi>, error out=w597:errorcluster)  [unwired: 1 in, 3 out]
            }
            frame 6 {
              n179 = control-ref of="path"() -> (w601:refnum<vi>)
              n180 = invoke class="VI" method="Ctrl Val.Set"(reference=w606, error in=w605, "Control Name"="path" ("控件名"), "Value"=w601) -> (reference out=w604:refnum<vi>, error out=w603:errorcluster)  [unwired: 1 in, 3 out]
            }
            frame 7 {
              n181 = Unbundle By Name(w608) -> ("chk1"=w607:bool)
              n182 = invoke class="VI" method="Ctrl Val.Set"(reference=w613, error in=w612, "Control Name"="check1" ("控件名"), "Value"=w607) -> (reference out=w611:refnum<vi>, error out=w610:errorcluster)  [unwired: 1 in, 3 out]
            }
            frame 8 {
              n183 = Unbundle By Name(w615) -> ("highspd"=w614:bool)
              n184 = invoke class="VI" method="Ctrl Val.Set"(reference=w620, error in=w619, "Control Name"="highspd" ("控件名"), "Value"=w614) -> (reference out=w618:refnum<vi>, error out=w617:errorcluster)  [unwired: 1 in, 3 out]
            }
            frame 9 {
              n185 = Unbundle By Name(w622) -> ("disp"=w621:bool)
              n186 = invoke class="VI" method="Ctrl Val.Set"(reference=w627, error in=w626, "Control Name"="disp" ("控件名"), "Value"=w621) -> (reference out=w625:refnum<vi>, error out=w624:errorcluster)  [unwired: 1 in, 3 out]
            }
            frame 10 {
              n187 = Unbundle By Name(w629) -> ("save"=w628:bool)
              n188 = invoke class="VI" method="Ctrl Val.Set"(reference=w634, error in=w633, "Control Name"="save" ("控件名"), "Value"=w628) -> (reference out=w632:refnum<vi>, error out=w631:errorcluster)  [unwired: 1 in, 3 out]
            }
            frame 11 {
              n189 = local read "reciveEnable"() -> (w635:bool)
              n190 = invoke class="VI" method="Ctrl Val.Set"(reference=w640, error in=w639, "Control Name"="Enable" ("控件名"), "Value"=w635) -> (reference out=w638:refnum<vi>, error out=w637:errorcluster)  [unwired: 1 in, 3 out]
            }
            frame 12 {
              n191 = control-ref of="SaveCnt"() -> (w641:refnum<vi>)
              n192 = invoke class="VI" method="Ctrl Val.Set"(reference=w646, error in=w645, "Control Name"="SaveCnt" ("控件名"), "Value"=w641) -> (reference out=w644:refnum<vi>, error out=w643:errorcluster)  [unwired: 1 in, 3 out]
            }
            frame 13 {
              n193 = invoke class="VI" method="Ctrl Val.Set"(reference=w652, error in=w651, "Control Name"="UseFilter" ("控件名"), "Value"=w647) -> (reference out=w650:refnum<vi>, error out=w649:errorcluster)  [unwired: 1 in, 3 out]
            }
            frame 14 {
              n194 = invoke class="VI" method="Ctrl Val.Set"(reference=w658, error in=w657, "Control Name"="Filter" ("控件名"), "Value"=w653) -> (reference out=w656:refnum<vi>, error out=w655:errorcluster)  [unwired: 1 in, 3 out]
            }
            frame 15 {
              n195 = Unbundle By Name(w660) -> ("ID合并"=w659:bool)
              n196 = invoke class="VI" method="Ctrl Val.Set"(reference=w665, error in=w664, "Control Name"="ID合并" ("控件名"), "Value"=w659) -> (reference out=w663:refnum<vi>, error out=w662:errorcluster)  [unwired: 1 in, 3 out]
            }
            frame 16 {
              n197 = control-ref of="errcnt2"() -> (w669:refnum<vi>)
              n198 = invoke class="VI" method="Ctrl Val.Set"(reference=w670, error in=w668, "Control Name"="errcnt2" ("控件名"), "Value"=w669) -> (reference out=w667:refnum<vi>, error out=w666:errorcluster)  [unwired: 1 in, 3 out]
            }
            frame 17 {
              n199 = control-ref of="Rrate2"() -> (w672:refnum<vi>)
              n200 = invoke class="VI" method="Ctrl Val.Set"(reference=w677, error in=w676, "Control Name"="rate1" ("控件名"), "Value"=w672) -> (reference out=w675:refnum<vi>, error out=w674:errorcluster)  [unwired: 1 in, 3 out]
            }
            frame 18 {
              n201 = control-ref of="Trate1"() -> (w678:refnum<vi>)
              n202 = invoke class="VI" method="Ctrl Val.Set"(reference=w683, error in=w682, "Control Name"="rate2" ("控件名"), "Value"=w678) -> (reference out=w681:refnum<vi>, error out=w680:errorcluster)  [unwired: 1 in, 3 out]
            }
            frame 19 {
              n203 = control-ref of="Trate2"() -> (w684:refnum<vi>)
              n204 = invoke class="VI" method="Ctrl Val.Set"(reference=w689, error in=w688, "Control Name"="rate3" ("控件名"), "Value"=w684) -> (reference out=w687:refnum<vi>, error out=w686:errorcluster)  [unwired: 1 in, 3 out]
            }
            frame 20 {
              n205 = Unbundle By Name(w691) -> ("chk2"=w690:bool)
              n206 = invoke class="VI" method="Ctrl Val.Set"(reference=w696, error in=w695, "Control Name"="check2" ("控件名"), "Value"=w690) -> (reference out=w694:refnum<vi>, error out=w693:errorcluster)  [unwired: 1 in, 3 out]
            }
            frame 21 {
              n207 = Unbundle By Name(w698) -> ("rateR1"=w697:bool)
              n208 = invoke class="VI" method="Ctrl Val.Set"(reference=w703, error in=w702, "Control Name"="Rrate1" ("控件名"), "Value"=w697) -> (reference out=w701:refnum<vi>, error out=w700:errorcluster)  [unwired: 1 in, 3 out]
            }
            frame 22 {
              n209 = Unbundle By Name(w705) -> ("rateR2"=w704:bool)
              n210 = invoke class="VI" method="Ctrl Val.Set"(reference=w710, error in=w709, "Control Name"="Rrate2" ("控件名"), "Value"=w704) -> (reference out=w708:refnum<vi>, error out=w707:errorcluster)  [unwired: 1 in, 3 out]
            }
            frame 23 {
              n211 = Unbundle By Name(w712) -> ("rateT1"=w711:bool)
              n212 = invoke class="VI" method="Ctrl Val.Set"(reference=w717, error in=w716, "Control Name"="Trate1" ("控件名"), "Value"=w711) -> (reference out=w715:refnum<vi>, error out=w714:errorcluster)  [unwired: 1 in, 3 out]
            }
            frame 24 {
              n213 = Unbundle By Name(w719) -> ("rateT2"=w718:bool)
              n214 = invoke class="VI" method="Ctrl Val.Set"(reference=w724, error in=w723, "Control Name"="Trate2" ("控件名"), "Value"=w718) -> (reference out=w722:refnum<vi>, error out=w721:errorcluster)  [unwired: 1 in, 3 out]
            }
            frame 26 {
              n215 = Unbundle By Name(w726) -> ("TSFormat"=w725:enum16{"原始值", "实际值"})
              n216 = invoke class="VI" method="Ctrl Val.Set"(reference=w731, error in=w730, "Control Name"="TSFormat" ("控件名"), "Value"=w725) -> (reference out=w729:refnum<vi>, error out=w728:errorcluster)  [unwired: 1 in, 3 out]
            }
            frame 27 {
              n217 = Unbundle By Name(w733) -> ("BuffLen"=w732:u16)
              n218 = invoke class="VI" method="Ctrl Val.Set"(reference=w738, error in=w737, "Control Name"="BuffLen" ("控件名"), "Value"=w732) -> (reference out=w736:refnum<vi>, error out=w735:errorcluster)  [unwired: 1 in, 3 out]
            }
            frame 25 {
              w739 = FALSE ("结束前等待")
              n219 = invoke class="VI" method="Run VI"(reference=w743, error in=w742, "Wait until done"=w739, "Auto Dispose Ref"=w739) -> (reference out=w741:refnum<vi>, error out=w740:errorcluster)  [unwired: 1 in, 3 out]
            }
          }
        }
        n220 = global write "_USB_CAN_GLOBAL_.vi" "open"(FALSE ("open")) -> ()
        n221 = Close Reference(reference=w423, error in (no error)=w422) -> ()  [unwired: 1 out]
        n222 = global write "_USB_CAN_GLOBAL_.vi" "close"(TRUE ("open")) -> ()
        n223 = Create User Event(user event datatype=w453) -> (user event=w451:refnum<user-event>)  [unwired: 1 in, 1 out]
        n224 = for {
          N: 12 -> [_]
          tunnel: w451 -> [w474]
          shift-right: [w477] -> w444
          shift-left: w458 -> [w478]
          shift-right: [w475] -> w419
          shift-left: w457 -> [w476]
          tunnel: w432 -> [w473]
          i -> [w479]
          n225 = case shown="0" w479 {
            tunnel: w478 -> [w481 w485 w490 w496 w502 w508 w514 w520 w527 w534 w541 w549 w555]
            tunnel: [w481 w482 w487 w493 w499 w505 w511 w517 w524 w531 w538 w546 w552] -> w477
            tunnel: w476 -> [w480 w484 w489 w495 w501 w507 w513 w519 w526 w533 w540 w548 w554]
            tunnel: [w480 w483 w488 w494 w500 w506 w512 w518 w525 w532 w539 w547 w553] -> w475
            tunnel: w474 -> [_ _ w486 _ _ _ _ _ _ _ _ _ _]
            tunnel: w473 -> [_ _ _ _ _ _ _ w516 _ _ _ _ _]
            frame -1, Default {
            }
            frame 0 {
              n226 = invoke class="VI" method="Default Vals.Reinit All"(reference=w485, error in=w484) -> (reference out=w482:refnum<vi>, error out=w483:errorcluster)  [unwired: 1 in, 1 out]
            }
            frame 1 {
              n227 = invoke class="VI" method="Ctrl Val.Set"(reference=w490, error in=w489, "Control Name"="event" ("控件名"), "Value"=w486) -> (reference out=w487:refnum<vi>, error out=w488:errorcluster)  [unwired: 1 in, 3 out]
            }
            frame 2 {
              n228 = local read "sendcycle"() -> (w492:i32)
              n229 = invoke class="VI" method="Ctrl Val.Set"(reference=w496, error in=w495, "Control Name"="Cycle" ("控件名"), "Value"=w492) -> (reference out=w493:refnum<vi>, error out=w494:errorcluster)  [unwired: 1 in, 3 out]
            }
            frame 3 {
              n230 = local read "SendCnt"() -> (w498:i32)
              n231 = invoke class="VI" method="Ctrl Val.Set"(reference=w502, error in=w501, "Control Name"="FrameCnt" ("控件名"), "Value"=w498) -> (reference out=w499:refnum<vi>, error out=w500:errorcluster)  [unwired: 1 in, 3 out]
            }
            frame 4 {
              n232 = local read "ID Inc"() -> (w504:bool)
              n233 = invoke class="VI" method="Ctrl Val.Set"(reference=w508, error in=w507, "Control Name"="ID Inc" ("控件名"), "Value"=w504) -> (reference out=w505:refnum<vi>, error out=w506:errorcluster)  [unwired: 1 in, 3 out]
            }
            frame 5 {
              n234 = local read "Data Inc"() -> (w510:bool)
              n235 = invoke class="VI" method="Ctrl Val.Set"(reference=w514, error in=w513, "Control Name"="Data Inc" ("控件名"), "Value"=w510) -> (reference out=w511:refnum<vi>, error out=w512:errorcluster)  [unwired: 1 in, 3 out]
            }
            frame 10 {
              n236 = invoke class="VI" method="Ctrl Val.Set"(reference=w520, error in=w519, "Control Name"="TFun" ("控件名"), "Value"=w516) -> (reference out=w517:refnum<vi>, error out=w518:errorcluster)  [unwired: 1 in, 3 out]
            }
            frame 6 {
              n237 = local read "Frame ID"() -> (w523:string)
              n238 = call "FormatIDString.vi"("ID String"=w523) -> ("ID"=w522:u32)
              n239 = invoke class="VI" method="Ctrl Val.Set"(reference=w527, error in=w526, "Control Name"="ID" ("控件名"), "Value"=w522) -> (reference out=w524:refnum<vi>, error out=w525:errorcluster)  [unwired: 1 in, 3 out]
            }
            frame 7 {
              n240 = local read "Frame Format"() -> (w530:u16)
              n241 = Not Equal To 0?(x=w530) -> (x != 0?=w529:bool)
              n242 = invoke class="VI" method="Ctrl Val.Set"(reference=w534, error in=w533, "Control Name"="ExtFrame" ("控件名"), "Value"=w529) -> (reference out=w531:refnum<vi>, error out=w532:errorcluster)  [unwired: 1 in, 3 out]
            }
            frame 8 {
              n243 = local read "Frame Type"() -> (w537:u16)
              n244 = Not Equal To 0?(x=w537) -> (x != 0?=w536:bool)
              n245 = invoke class="VI" method="Ctrl Val.Set"(reference=w541, error in=w540, "Control Name"="remote" ("控件名"), "Value"=w536) -> (reference out=w538:refnum<vi>, error out=w539:errorcluster)  [unwired: 1 in, 3 out]
            }
            frame 9 {
              n246 = local read "data"() -> (w544:string)
              n247 = call "str_to_u32_arr.vi"("string"=w544) -> ("array"=w545:u32[])
              n248 = To Unsigned Byte Integer(number=w545) -> (unsigned 8bit integer=w543:u8[])
              n249 = invoke class="VI" method="Ctrl Val.Set"(reference=w549, error in=w548, "Control Name"="data" ("控件名"), "Value"=w543) -> (reference out=w546:refnum<vi>, error out=w547:errorcluster)  [unwired: 1 in, 3 out]
            }
            frame 11 {
              w551 = FALSE ("结束前等待")
              n250 = invoke class="VI" method="Run VI"(reference=w555, error in=w554, "Wait until done"=w551, "Auto Dispose Ref"=w551) -> (reference out=w552:refnum<vi>, error out=w553:errorcluster)  [unwired: 1 in, 3 out]
            }
          }
        }
        n251 = disable-structure shown="启用" {
          disable-tunnel: [" - 设备未启动" ("字符串") w471] -> w415
          frame Disabled {
          }
          frame Enabled {
            n252 = call "sub-Language-get str-const.vi"("sid"=u32 512) -> ("str"=w471:string)
          }
        }
        n253 = Create User Event(user event datatype=w434) -> (user event=w433:refnum<user-event>)  [unwired: 1 in, 1 out]
        n254 = register-events(w451, w446, w433) -> (reference out=w452:refnum<event-registration>)  [unwired: 2 in, 1 out]
        n255 = Unbundle By Name(w421) -> ("autoconn"=w420:bool)
        n256 = Concatenate Strings(w413, w415) -> (w414:string)
        n257 = property class="VI"("Front Panel.Title"=w414) -> ()  [unwired: 2 in, 2 out]
        n258 = property on="send stop" class="Bool (严格)"("Val(Sgnl)"=TRUE ("值(信号)")) -> ()  [unwired: 2 in, 2 out]
        n259 = case shown="真" w420 {
          tunnel: w419 -> [_ _]
          tunnel: w418 -> [_ _]
          frame False {
          }
          frame True {
            n260 = call "important information-autoConn1.vi"() -> ()  [unwired: 12 in]
          }
        }
      }
      frame "run" {
        n261 = event shown="[3] 菜单选择(用户)" {
          selector: w758 -> [_ _ _ _ _ _ _ _ _ _ _ _ _ _ _ _ _ _ _ _ _]
          dyn-events: [_ _ _ _ _ _ _ _ _ _ _ _ _ _ _ _ _ _ _ _ _] -> w757
          timeout: 100 -> [_ _ _ _ _ _ _ _ _ _ _ _ _ _ _ _ _ _ _ _ _]
          tunnel: w785 -> [w810 w851 w869 w884 _ w1948 w1952 w2013 w2036 w2060 w2065 w2150 w2174 w2196 w2220 w2236 w2252 w2269 w2285 w2301 w2331]
          tunnel: w784 -> [w809 w850 w868 w898 w1867 w1947 w1965 w2012 w2035 w2059 w2077 w2149 w2173 w2195 w2219 w2235 w2251 w2268 w2284 _ w2316]
          tunnel: w783 -> [w808 w849 w867 w897 w1866 w1946 w1964 w2011 w2034 w2058 w2076 w2148 w2172 w2194 w2218 w2234 w2250 w2267 _ w2300 w2330]
          tunnel: w782 -> [w807 w848 w866 w896 w1865 w1945 w1963 w2010 w2033 w2057 w2067 w2147 w2171 w2193 w2217 w2233 w2249 _ w2283 w2299 w2329]
          tunnel: w781 -> [w806 w847 w865 w885 w1858 w1944 w1949 w2009 w2032 w2056 w2061 w2146 w2170 w2192 w2216 w2232 _ w2266 w2282 w2298 w2328]
          tunnel: w780 -> [w805 w846 w864 w895 w1864 w1943 w1962 w2008 w2031 w2055 w2075 w2145 w2163 _ w2215 w2231 w2248 w2265 w2281 w2297 w2327]
          tunnel: w779 -> [w804 w845 w863 w894 w1863 w1942 w1961 w2007 w2030 w2054 w2074 w2144 w2166 w2180 w2214 w2230 w2247 w2264 w2280 w2296 w2326]
          tunnel: w778 -> [w803 w844 w862 w893 w1862 w1941 w1960 w2006 w2029 w2053 w2069 w2143 w2169 w2191 _ w2229 w2246 w2263 w2279 w2295 w2325]
          tunnel: w777 -> [w802 w843 w861 w892 w1861 w1940 w1959 w2005 w2028 w2052 w2068 w2142 w2168 w2190 w2213 _ w2245 w2262 w2278 w2294 w2324]
          tunnel: [w810 w851 w869 w883 w1857 w1948 w1952 w2013 w2036 w2060 w2065 w2150 w2174 w2196 w2220 w2236 w2252 w2269 w2285 w2301 w2331] -> w776
          tunnel: [w809 w850 w868 w898 w1867 w1947 w1965 w2012 w2035 w2059 w2077 w2149 w2173 w2195 w2219 w2235 w2251 w2268 w2284 w2292 w2316] -> w775
          tunnel: [w808 w849 w867 w897 w1866 w1946 w1964 w2011 w2034 w2058 w2076 w2148 w2172 w2194 w2218 w2234 w2250 w2267 w2276 w2300 w2330] -> w774
          tunnel: [w807 w848 w866 w896 w1865 w1945 w1963 w2010 w2033 w2057 w2067 w2147 w2171 w2193 w2217 w2233 w2249 w2259 w2283 w2299 w2329] -> w773
          tunnel: [w806 w847 w865 w885 w1858 w1944 w1949 w2009 w2032 w2056 w2061 w2146 w2170 w2192 w2216 w2232 w2243 w2266 w2282 w2298 w2328] -> w772
          tunnel: [w805 w846 w864 w895 w1864 w1943 w1962 w2008 w2031 w2055 w2075 w2145 w2163 w2178 w2215 w2231 w2248 w2265 w2281 w2297 w2327] -> w771
          tunnel: [w804 w845 w863 w894 w1863 w1942 w1961 w2007 w2030 w2054 w2074 w2144 w2161 w2180 w2214 w2230 w2247 w2264 w2280 w2296 w2326] -> w770
          tunnel: [w803 w844 w862 w893 w1862 w1941 w1960 w2006 w2029 w2053 w2069 w2143 w2169 w2191 w2206 w2229 w2246 w2263 w2279 w2295 w2325] -> w769
          tunnel: [w802 w843 w861 w892 w1861 w1940 w1959 w2005 w2028 w2052 w2068 w2142 w2168 w2190 w2213 w2227 w2245 w2262 w2278 w2294 w2324] -> w768
          tunnel: [T1."run" T1."run" T1."run" T1."run" T1."run" T1."unRegistEvent" T1."run" T1."run" T1."run" T1."run" T1."run" T1."run" T1."run" T1."run" T1."run" T1."run" T1."run" T1."run" T1."run" T1."run" T1."run"] -> w767
          tunnel: w766 -> [w800 w841 w859 w890 w1859 w1938 w1957 w2003 w2026 w2050 _ _ w2165 w2183 w2211 w2226 w2242 w2258 w2275 w2291 w2322]
          tunnel: [w800 w841 w859 w890 w1859 w1938 w1957 w2003 w2026 w2050 TRUE FALSE w2165 w2183 w2211 w2226 w2242 w2258 w2275 w2291 w2322] -> w765
          tunnel: w752 -> [_ _ _ w881 _ _ _ w1993 _ _ _ _ _ _ _ _ _ _ _ _ _]
          tunnel: w764 -> [w799 w840 w858 w889 w1848 w1936 w1956 w2002 w2025 w2049 w2071 w2137 w2164 w2182 w2210 w2225 w2241 w2257 w2274 w2290 w2321]
          tunnel: [w799 w840 w858 w888 w1848 w1936 w1956 w2002 w2025 w2049 w2071 w2137 w2164 w2182 w2210 w2225 w2241 w2257 w2274 w2290 w2321] -> w763
          tunnel: w762 -> [_ w838 _ w882 _ _ _ w1996 w2024 w2048 _ _ w2156 w2181 _ _ _ _ _ _ _]
          tunnel: w761 -> [_ _ _ w871 _ _ w1954 _ _ _ w2070 w2134 _ _ _ _ _ _ _ _ _]
          tunnel: w760 -> [w798 w832 w857 w887 w1852 w1935 w1955 w2001 w2023 w2047 w2066 w2136 w2160 w2179 w2209 w2224 w2240 w2256 w2273 w2289 w2320]
          tunnel: [w798 w832 w857 w886 w1850 w1935 w1955 w2001 w2023 w2047 w2066 w2136 w2160 w2179 w2209 w2224 w2240 w2256 w2273 w2289 w2320] -> w759
          tunnel: w756 -> [_ _ _ _ _ _ _ _ _ _ _ _ _ _ _ _ _ _ _ _ _]
          tunnel: w754 -> [w792 w837 w854 w879 w1851 w1934 w1953 w1995 w2022 w2046 w2064 w2133 w2154 w2177 w2205 w2223 w2239 w2255 w2272 w2288 w2319]
          tunnel: [w792 w835 w854 w878 w1851 w1934 w1953 w1994 w2022 w2046 w2064 w2133 w2154 w2177 w2205 w2223 w2239 w2255 w2272 w2288 w2319] -> w753
          tunnel: w751 -> [w797 w834 w853 w877 w1856 w1933 w1951 w2000 w2021 w2045 w2063 w2132 w2153 w2176 w2204 w2222 w2238 w2254 w2271 w2287 w2318]
          tunnel: [w797 w834 w853 w876 w1856 w1933 w1951 w2000 w2021 w2045 w2063 w2132 w2153 w2176 w2204 w2222 w2238 w2254 w2271 w2287 w2318] -> w750
          tunnel: w749 -> [w789 _ _ w875 _ _ _ _ _ _ _ _ _ _ _ _ _ _ _ _ _]
          tunnel: w748 -> [w796 w833 w852 w874 w1845 w1932 w1950 w1999 w2020 w2044 w2062 w2131 w2152 w2175 w2203 w2221 w2237 w2253 w2270 w2286 w2317]
          tunnel: [w796 w833 w852 w873 w1849 w1932 w1950 w1999 w2020 w2044 w2062 w2131 w2152 w2175 w2203 w2221 w2237 w2253 w2270 w2286 w2317] -> w747
          tunnel: w746 -> [w786 _ _ w872 w1854 _ _ _ _ _ _ _ _ _ _ _ _ _ _ _ _]
          tunnel: w745 -> [_ _ _ w870 _ _ _ _ _ _ _ _ _ _ _ _ _ _ _ _ _]
          event Timeout {
            n262 = event-data() -> ()  [unwired: 1 in, 1 out]
            n263 = Unbundle By Name(w792) -> ("autoconn"=w791:bool)
            n264 = global read "_USB_CAN_GLOBAL_.vi" "open"() -> (w788:bool)
            n265 = global read "_USB_CAN_GLOBAL_.vi" "close"() -> (w787:bool)
            n266 = feedback-in #1(w788) -> ()
            n267 = feedback #1(FALSE ("open")) -> (w794:bool)
            n268 = Compound Arithmetic op=AND(invert w788, w791, invert w787) -> (w790:bool)
            n269 = Compound Arithmetic op=AND(w794, invert w788) -> (w793:bool)
            n270 = case shown="真" w793 {
              tunnel: w786 -> [_ w830]
              frame False {
              }
              frame True {
                n271 = call "sub-Language-get str-const.vi"("sid"=u32 265) -> ("str"=w827:string)
                n272 = Concatenate Strings(w830, " - " ("字符串"), w827) -> (w829:string)
                n273 = property class="VI"("Front Panel.Title"=w829) -> ()  [unwired: 2 in, 2 out]
              }
            }
            n274 = case shown="真" w790 {
              tunnel: w789 -> [_ w816]
              tunnel: w786 -> [_ w813]
              frame False {
              }
              frame True {
                n275 = Tick Count (ms)() -> (millisecond timer value=w818:u32)
                n276 = call "sub-Language-get str-const.vi"("sid"=u32 265) -> ("str"=w811:string)
                n277 = feedback #2(w818) -> (w819:u32)
                n278 = Concatenate Strings(w813, " - " ("字符串"), w811) -> (w815:string)
                n279 = Subtract(x=w818, y=w819) -> (x-y=w822:u32)
                n280 = property class="VI"("Front Panel.Title"=w815) -> ()  [unwired: 2 in, 2 out]
                n281 = Greater?(x=w822, y=u32 1000) -> (0:w820:bool)
                n282 = case shown="真" w820 {
                  tunnel: w819 -> [w823 _]
                  tunnel: w818 -> [_ w826]
                  tunnel: [w823 w826] -> w817
                  tunnel: w816 -> [_ w824]
                  frame False {
                  }
                  frame True {
                    n283 = Generate User Event(user event=w824, event data cluster=FALSE ("事件数据")) -> ()  [unwired: 1 in, 2 out]
                  }
                }
                n284 = feedback-in #2(w817) -> ()
              }
            }
          }
          event User Event {
            w836 = FALSE
            # "123"
            n285 = event-data() -> ()  [unwired: 1 in, 1 out]
            n286 = invoke class="VI" method="Ctrl Val.Set"(reference=w838, "Control Name"="save" ("控件名"), "Value"=w836) -> ()  [unwired: 2 in, 5 out]
            n287 = Bundle By Name(cluster=w837, "save"=w836) -> (w835:T2)
          }
          event User Event {
            w855 = T4."Enabled" ("禁用")
            n288 = event-data() -> ()  [unwired: 1 in, 1 out]
            n289 = property on="send stop" class="Bool (严格)"("DisabledEnum"=T4."Disabled and Grayed Out" ("禁用")) -> ()  [unwired: 2 in, 2 out]
            n290 = property on="Send" class="Bool"("DisabledEnum"=w855) -> ()  [unwired: 2 in, 2 out]
            n291 = property on="data" class="Str"("DisabledEnum"=w855) -> ()  [unwired: 2 in, 2 out]
            n292 = property on="ID Inc" class="Bool (严格)"("DisabledEnum"=w855) -> ()  [unwired: 2 in, 2 out]
            n293 = property on="sendcycle" class="DigNum (严格)"("DisabledEnum"=w855) -> ()  [unwired: 2 in, 2 out]
            n294 = property on="Data Inc" class="Bool (严格)"("DisabledEnum"=w855) -> ()  [unwired: 2 in, 2 out]
            n295 = property on="SendCnt" class="DigNum (严格)"("DisabledEnum"=w855) -> ()  [unwired: 2 in, 2 out]
          }
          event Menu Selection (User) {
            n296 = event-data() -> ("ItemTag"=w880:string)  [unwired: 1 in]
            n297 = case shown="\"\", 默认" w880 {
              selector: w880 -> [w901 _ _ _ _ _ _ _ _ _ w1283 w1307 w1330 w1351 w1373 w1394 w1410 w1430 _ _ _ w1543 w1557 w1569 w1592 w1614 w1630 w1653 w1722 w1746 w1766 w1790 _ _ w1828]
              tunnel: w889 -> [w912 _ _ w1026 w1043 w1090 w1136 w1182 w1217 w1233 w1297 w1321 w1343 w1354 w1379 w1400 w1416 w1436 w1444 w1487 w1515 w1548 w1562 w1574 w1596 w1618 w1635 w1664 w1728 w1752 w1772 w1796 w1805 w1817 w1836]
              tunnel: [w912 u16 3 u16 4 w1026 w1043 w1090 w1136 w1182 w1217 w1233 w1297 w1321 w1343 w1354 w1379 w1400 w1416 w1436 w1444 w1487 w1515 w1548 w1562 w1574 w1596 w1618 w1635 w1664 w1728 w1752 w1772 w1796 w1805 w1817 w1836] -> w888
              tunnel: w887 -> [w911 w980 w1016 w1025 w1045 w1092 w1138 w1184 w1220 w1235 w1299 w1323 w1345 w1352 w1377 w1398 w1414 w1434 w1445 w1494 w1517 w1547 w1561 w1573 w1595 w1617 w1634 w1663 w1726 w1750 w1770 w1794 w1804 w1816 w1835]
              tunnel: [w911 w980 w1016 w1025 w1045 w1092 w1138 w1184 w1220 w1234 w1299 w1323 w1345 w1352 w1377 w1398 w1414 w1434 w1445 w1494 w1517 w1547 w1561 w1573 w1595 w1617 w1634 w1663 w1726 w1750 w1770 w1794 w1804 w1816 w1835] -> w886
              tunnel: w885 -> [_ _ _ _ _ _ _ _ _ _ _ _ _ _ _ _ _ _ _ _ _ _ _ _ _ _ _ _ _ _ _ _ _ _ _]
              tunnel: w884 -> [w910 w979 w1015 w1022 w1044 w1091 w1137 w1183 w1216 w1236 w1298 w1322 w1344 w1353 w1378 w1399 w1415 w1435 w1447 w1500 w1516 w1546 w1560 w1572 w1594 w1616 w1633 w1662 w1727 w1751 w1771 w1795 w1803 w1815 w1834]
              tunnel: [w910 w979 w1015 w1022 w1039 w1087 w1133 w1179 w1216 w1236 w1298 w1322 w1344 w1353 w1378 w1399 w1415 w1435 w1447 w1500 w1516 w1546 w1560 w1572 w1594 w1616 w1633 w1662 w1727 w1751 w1771 w1795 w1803 w1815 w1834] -> w883
              tunnel: w881 -> [w902 w976 w1010 _ _ _ _ _ _ _ w1285 w1308 w1332 w1350 w1374 w1395 w1411 w1431 _ _ _ w1545 w1559 w1571 w1593 w1615 w1632 w1642 w1723 w1747 w1767 w1791 _ _ _]
              tunnel: w882 -> [_ _ _ w1019 w1038 _ _ _ _ _ _ _ w1334 _ w1372 w1393 _ _ _ _ _ w1541 w1555 _ w1580 w1602 w1628 w1651 w1721 w1745 w1765 w1789 _ _ _]
              tunnel: w879 -> [w909 w963 w999 w1024 w1041 w1089 w1135 w1181 w1219 w1229 w1292 w1318 w1340 w1348 w1369 w1385 w1408 w1419 w1446 w1499 w1518 w1539 w1552 w1567 w1591 w1613 w1626 w1661 w1718 w1730 w1762 w1774 w1802 w1814 w1833]
              tunnel: [w909 w973 w1009 w1024 w1041 w1089 w1135 w1181 w1219 w1229 w1291 w1317 w1339 w1347 w1370 w1391 w1409 w1429 w1446 w1499 w1518 w1538 w1551 w1566 w1590 w1612 w1624 w1660 w1719 w1743 w1763 w1787 w1802 w1814 w1833] -> w878
              tunnel: w877 -> [w908 w971 w1007 _ _ _ _ _ w1221 w1232 w1296 w1320 w1342 w1355 w1368 w1390 w1407 w1428 w1448 w1497 w1514 w1537 w1550 w1565 w1589 w1611 w1623 w1659 w1717 w1742 w1761 w1786 w1801 w1813 w1832]
              tunnel: [w908 w971 w1007 TRUE w1039 w1087 w1133 w1179 w1221 w1232 w1296 w1320 w1342 w1355 w1368 w1390 w1407 w1428 w1448 w1497 w1514 w1537 w1550 w1565 w1589 w1611 w1623 w1659 w1717 w1742 w1761 w1786 w1801 w1813 w1832] -> w876
              tunnel: w875 -> [_ _ _ w1021 _ _ _ _ _ _ _ _ _ _ _ _ _ _ _ _ _ _ _ _ _ _ _ _ _ _ _ _ _ _ _]
              tunnel: w874 -> [w907 w970 w1006 _ _ _ _ _ _ w1231 w1295 w1319 w1341 w1356 w1367 w1389 w1406 w1427 w1449 w1498 w1513 w1536 w1549 w1564 w1588 w1610 w1622 w1658 w1716 w1741 w1760 w1785 w1800 w1812 w1831]
              tunnel: [w907 w970 w1006 _ _ _ _ _ _ w1231 w1295 w1319 w1341 w1356 w1367 w1389 w1406 w1427 w1449 w1498 w1513 w1536 w1549 w1564 w1588 w1610 w1622 w1658 w1716 w1741 w1760 w1785 w1800 w1812 w1831] -> w873
              tunnel: w872 -> [w900 _ _ _ w1040 w1088 w1134 w1180 _ _ _ _ _ _ _ _ _ _ _ _ _ _ _ _ _ _ _ _ _ _ _ _ _ _ _]
              tunnel: w871 -> [_ _ _ _ w1037 _ _ _ _ w1228 _ _ _ _ _ _ _ _ _ _ _ _ _ _ _ _ _ _ _ _ _ _ _ _ _]
              tunnel: w870 -> [_ _ _ _ _ _ _ _ _ _ _ _ _ _ _ _ _ _ _ _ _ _ _ _ _ _ _ _ _ _ _ _ w1797 _ _]
              frame "", Default {
                n298 = local read "selected"() -> (w899:i32)
                n299 = Scan From String(format string="L%04d" ("格式字符串"), input string=w901, default 1=0 ("默认值 1")) -> (error out=w905:errorcluster, output 1=w904:i32)  [unwired: 2 in, 2 out]
                n300 = case shown="无错误" w905 {
                  tunnel: w904 -> [w913 _]
                  tunnel: w902 -> [w917 _]
                  tunnel: w899 -> [w920 _]
                  tunnel: w900 -> [w916 _]
                  frame No Error {
                    n301 = global read "sub-Language global.vi" "languages"() -> (w914:T6)
                    n302 = Not Equal?(x=w913, y=w920) -> (x != y?=w919:bool)
                    n303 = local write "selected"(w913) -> ()
                    n304 = call "sub-SetLanguageSel.vi"("sel"=w913) -> ()  [unwired: 11 in]
                    n305 = Array Size(array=w914) -> (size(s)=w921:i32)
                    n306 = for {
                      N: w921 -> [_]
                      tunnel: w917 -> [w950]
                      tunnel: w913 -> [w946]
                      tunnel: [w944] -> w915
                      i -> [w947]
                      n307 = Equal?(x=w947, y=w946) -> (x = y?=w945:bool)
                      n308 = Format Into String(format string="L%04d" ("格式字符串"), w947) -> (resulting string=w948:string)  [unwired: 2 in, 1 out]
                      n309 = Set Menu Item Info(6:w945, 7:w948, 11:w950) -> (0:w944:errorcluster)  [unwired: 4 in, 1 out]
                    }
                    n310 = global read "sub-Language global.vi" "menu items"() -> (w918:string[])
                    n311 = case shown="真" w919 {
                      tunnel: w918 -> [_ w927]
                      tunnel: w917 -> [_ w926]
                      tunnel: w916 -> [_ w923]
                      tunnel: w915 -> [_ _]
                      tunnel: w914 -> [_ w925]
                      tunnel: w913 -> [_ w924]
                      frame False {
                      }
                      frame True {
                        n312 = stacked-sequence {
                          tunnel: w927 -> [_ w931 _]
                          tunnel: w926 -> [_ w930 w942]
                          tunnel: w925 -> [w929 _ _]
                          tunnel: w924 -> [w928 _ _]
                          tunnel: w923 -> [_ _ w939]
                          tunnel: [_ _ w938] -> w922
                          frame #0 {
                            n313 = call "sub-Language load.vi"("selected"=w928, "languages"=w929) -> ()  [unwired: 9 in, 1 out]
                          }
                          frame #1 {
                            n314 = for {
                              tunnel: w931 -> [w936] mode=indexing
                              tunnel: w930 -> [w937]
                              n315 = Scan From String(format string="m%x" ("格式字符串"), input string=w936, default 1=u32 0 ("默认值 1")) -> (output 1=w934:u32)  [unwired: 2 in, 3 out]
                              n316 = call-poly "sub-Language-get str.vi"("sid"=w934) -> ("str"=w932:string)
                              n317 = Set Menu Item Info(7:w936, 10:w932, 11:w937) -> ()  [unwired: 4 in, 2 out]
                            }
                          }
                          frame #2 {
                            n318 = control-ref of="本VI"() -> (w943:refnum<vi>)
                            n319 = call "sub-set menu short key.vi"("menubar in"=w942) -> ()  [unwired: 9 in, 2 out]
                            n320 = call "sub-Language-get str-const.vi"("sid"=u32 512) -> ("str"=w941:string)
                            n321 = call "sub-import vi String.vi"("vi ref"=w943) -> ()  [unwired: 10 in, 1 out]
                            n322 = Concatenate Strings(w939, w941) -> (w938:string)
                          }
                        }
                        n323 = property class="VI"("Front Panel.Title"=w922) -> ()  [unwired: 2 in, 2 out]
                      }
                    }
                  }
                  frame Error {
                  }
                }
              }
              frame "m0007" {
                w962 = 2
                w964 = FALSE ("已勾选")
                n324 = property on="CAN Channel" class="Ring (严格)"() -> ("Value"=w960:u16)  [unwired: 2 in, 2 out]
                n325 = Set Menu Item Info(6:TRUE ("已勾选"), 7:"m0007" ("项标识符"), 11:w976) -> (3:w975:refnum<k9>)  [unwired: 4 in, 1 out]
                n326 = Equal?(x=w960, y=enum16{"1", "2"}."2") -> (x = y?=w958:bool)
                n327 = case shown="真" w958 {
                  frame False {
                  }
                  frame True {
                    n328 = property on="CAN Channel" class="Ring (严格)"("Value"=enum16{"1", "2"}."1" ("CAN Channel")) -> ()  [unwired: 2 in, 2 out]
                  }
                }
                n329 = Set Menu Item Info(6:w964, 7:"m0008" ("项标识符"), 11:w975) -> (3:w965:refnum<k9>)  [unwired: 4 in, 1 out]
                n330 = Set Menu Item Info(7:"m0037" ("项标识符"), 9:w964, 11:w965) -> ()  [unwired: 4 in, 2 out]
                n331 = Set Menu Item Info(7:"m0027" ("项标识符"), 9:w964, 11:w965) -> ()  [unwired: 4 in, 2 out]
                n332 = Set Menu Item Info(7:"m002D" ("项标识符"), 9:w964, 11:w965) -> ()  [unwired: 4 in, 2 out]
                n333 = Set Menu Item Info(7:"m002F" ("项标识符"), 9:w964, 11:w965) -> ()  [unwired: 4 in, 2 out]
                n334 = Open VI Reference(vi path=path "DeviceOP/ReciveThread.vi" ("VI路径")) -> (vi reference=w954:refnum<vi>, error out=w956:errorcluster)  [unwired: 5 in]
                n335 = property on="errcnt2" class="DigNum (严格)"("DisabledEnum"=w962) -> ()  [unwired: 2 in, 2 out]
                n336 = property on="Trate2" class="DigNum (严格)"("DisabledEnum"=w962) -> ()  [unwired: 2 in, 2 out]
                n337 = property on="Rrate2" class="DigNum (严格)"("DisabledEnum"=w962) -> ()  [unwired: 2 in, 2 out]
                n338 = invoke class="VI" method="Ctrl Val.Set"(reference=w954, error in=w956, "Control Name"="Enable2" ("控件名"), "Value"=FALSE) -> (reference out=w952:refnum<vi>, error out=w951:errorcluster)  [unwired: 1 in, 3 out]
                n339 = property on="CAN Channel" class="Ring (严格)"("Disabled Items []"=i32[] [1] ("禁用项[]")) -> ()  [unwired: 2 in, 2 out]
                n340 = Close Reference(reference=w952, error in (no error)=w951) -> ()  [unwired: 1 out]
                n341 = Bundle By Name(cluster=w963, "type"=u16 3 ("devtype")) -> (w973:T2)
              }
              frame "m0008" {
                w992 = 2
                w993 = 0
                w1000 = TRUE ("已勾选")
                n342 = Set Menu Item Info(6:FALSE ("已勾选"), 7:"m0007" ("项标识符"), 11:w1010) -> (3:w1012:refnum<k9>)  [unwired: 4 in, 1 out]
                n343 = Unbundle By Name(w999) -> ("rateR2"=w998:bool, "rateT2"=w996:bool, "chk2"=w986:bool, "RcvE2"=w985:bool)
                n344 = Set Menu Item Info(6:w1000, 7:"m0008" ("项标识符"), 11:w1012) -> (3:w1001:refnum<k9>)  [unwired: 4 in, 1 out]
                n345 = Set Menu Item Info(7:"m0037" ("项标识符"), 9:w1000, 11:w1001) -> ()  [unwired: 4 in, 2 out]
                n346 = Set Menu Item Info(7:"m0027" ("项标识符"), 9:w1000, 11:w1001) -> ()  [unwired: 4 in, 2 out]
                n347 = Set Menu Item Info(7:"m002D" ("项标识符"), 9:w1000, 11:w1001) -> ()  [unwired: 4 in, 2 out]
                n348 = Set Menu Item Info(7:"m002F" ("项标识符"), 9:w1000, 11:w1001) -> ()  [unwired: 4 in, 2 out]
                n349 = Bundle By Name(cluster=w999, "type"=u16 4 ("devtype")) -> (w1009:T2)
                n350 = Select(t=w993, s=w996, f=w992) -> (s? t:f=w995:i32)
                n351 = Select(t=w993, s=w998, f=w992) -> (s? t:f=w997:i32)
                n352 = Select(t=w993, s=w986, f=w992) -> (s? t:f=w994:i32)
                n353 = property on="Trate2" class="DigNum (严格)"("DisabledEnum"=w995) -> ()  [unwired: 2 in, 2 out]
                n354 = property on="errcnt2" class="DigNum (严格)"("DisabledEnum"=w994) -> ()  [unwired: 2 in, 2 out]
                n355 = property on="Rrate2" class="DigNum (严格)"("DisabledEnum"=w997) -> ()  [unwired: 2 in, 2 out]
                n356 = property on="CAN Channel" class="Ring (严格)"("Disabled Items []"=i32[] [] ("禁用项[]")) -> ()  [unwired: 2 in, 2 out]
                n357 = Open VI Reference(vi path=path "DeviceOP/ReciveThread.vi" ("VI路径")) -> (vi reference=w989:refnum<vi>, error out=w987:errorcluster)  [unwired: 5 in]
                n358 = invoke class="VI" method="Ctrl Val.Set"(reference=w989, error in=w987, "Control Name"="Enable2" ("控件名"), "Value"=w985) -> (reference out=w984:refnum<vi>, error out=w983:errorcluster)  [unwired: 1 in, 3 out]
                n359 = Close Reference(reference=w984, error in (no error)=w983) -> ()  [unwired: 1 out]
              }
              frame "m0009" {
                n360 = global read "_USB_CAN_GLOBAL_.vi" "open"() -> (w1020:bool)
                n361 = case shown="真" w1020 {
                  tunnel: w1021 -> [w1031 _]
                  tunnel: w1019 -> [w1029 _]
                  frame False {
                    n362 = invoke class="VI" method="Ctrl Val.Set"(reference=w1029, "Control Name"="open" ("控件名"), "Value"=TRUE) -> ()  [unwired: 2 in, 5 out]
                    n363 = Generate User Event(user event=w1031, event data cluster=TRUE ("事件数据")) -> ()  [unwired: 1 in, 2 out]
                  }
                  frame True {
                    n364 = call "sub-Language-get str-const.vi"("sid"=u32 256) -> ("str"=w1034:string)
                    n365 = call "sub-Language-get str-const.vi"("sid"=u32 257) -> ("str"=w1032:string)
                    n366 = call "TimeLmtDialog.vi"("Infoin"=w1032, "title"=w1034) -> ()  [unwired: 10 in]
                  }
                }
                n367 = global write "_USB_CAN_GLOBAL_.vi" "close"(FALSE ("open")) -> ()
              }
              frame "m000A" {
                w1039 = FALSE
                n368 = case shown="真" w1044 {
                  tunnel: w1043 -> [_ w1053]
                  tunnel: w1038 -> [_ w1051]
                  tunnel: w1037 -> [_ w1050]
                  frame False {
                    n369 = call "sub-Language-get str-const.vi"("sid"=u32 256) -> ("str"=w1046:string)
                    n370 = call "sub-Language-get str-const.vi"("sid"=u32 258) -> ("str"=w1048:string)
                    n371 = call "TimeLmtDialog.vi"("Infoin"=w1048, "title"=w1046) -> ()  [unwired: 10 in]
                  }
                  frame True {
                    n372 = local read "DevIndex"() -> (w1052:u32)
                    n373 = stacked-sequence {
                      tunnel: w1053 -> [_ w1057 w1068]
                      tunnel: w1052 -> [_ w1056 w1067]
                      tunnel: w1051 -> [w1055 _ _]
                      tunnel: w1050 -> [w1054 _ _]
                      frame #0 {
                        n374 = call "PreCloseDevice.vi"("Send Thread"=w1054, "Update Thread"=w1055) -> ()  [unwired: 10 in]
                      }
                      frame #1 {
                        n375 = Equal?(x=w1057, y=u16 4) -> (x = y?=w1061:bool)
                        n376 = Select(t=2, s=w1061, f=1) -> (s? t:f=w1058:i32)
                        n377 = for {
                          N: w1058 -> [_]
                          tunnel: w1057 -> [w1065]
                          tunnel: w1056 -> [w1064]
                          i -> [w1063]
                          n378 = call "ResetCAN.vi"("CANInd"=w1063, "DeciceInd"=w1064, "DeviceType"=w1065) -> ()  [unwired: 7 in, 2 out]
                        }
                      }
                      frame #2 {
                        n379 = local write "brgsta"(u16 0 ("brgsta")) -> ()
                        n380 = call "CloseDevice.vi"("DeviceInd"=w1067, "type"=w1068) -> ("success"=w1069:bool)  [unwired: 8 in, 1 out]
                        n381 = case shown="真" w1069 {
                          frame False {
                            n382 = call "sub-Language-get str-const.vi"("sid"=u32 256) -> ("str"=w1072:string)
                            n383 = call "sub-Language-get str-const.vi"("sid"=u32 260) -> ("str"=w1070:string)
                            n384 = call "TimeLmtDialog.vi"("Infoin"=w1070, "title"=w1072) -> ()  [unwired: 10 in]
                          }
                          frame True {
                            n385 = call "sub-Language-get str-const.vi"("sid"=u32 259) -> ("str"=w1074:string)
                            n386 = call "sub-Language-get str-const.vi"("sid"=u32 256) -> ("str"=w1076:string)
                            n387 = call "TimeLmtDialog.vi"("Infoin"=w1074, "title"=w1076) -> ()  [unwired: 10 in]
                          }
                        }
                      }
                    }
                  }
                }
                n388 = global write "_USB_CAN_GLOBAL_.vi" "open"(FALSE ("open")) -> ()
                n389 = global write "_USB_CAN_GLOBAL_.vi" "close"(TRUE ("open")) -> ()
                n390 = property class="VI"("Front Panel.Title"=w1040) -> ()  [unwired: 2 in, 2 out]
              }
              frame "m000C" {
                w1087 = FALSE
                n391 = case shown="真" w1091 {
                  tunnel: w1090 -> [_ w1105]
                  tunnel: [_ w1103] -> w1078
                  frame False {
                  }
                  frame True {
                    n392 = local read "DevIndex"() -> (w1104:u32)
                    n393 = stacked-sequence {
                      tunnel: w1105 -> [w1107 w1118]
                      tunnel: w1104 -> [w1106 w1117]
                      tunnel: [_ w1116] -> w1103
                      frame #0 {
                        n394 = Equal?(x=w1107, y=u16 4) -> (x = y?=w1111:bool)
                        n395 = Select(t=2, s=w1111, f=1) -> (s? t:f=w1108:i32)
                        n396 = for {
                          N: w1108 -> [_]
                          tunnel: w1107 -> [w1115]
                          tunnel: w1106 -> [w1114]
                          i -> [w1113]
                          n397 = call "ResetCAN.vi"("CANInd"=w1113, "DeciceInd"=w1114, "DeviceType"=w1115) -> ()  [unwired: 7 in, 2 out]
                        }
                      }
                      frame #1 {
                        n398 = call "CloseDevice.vi"("DeviceInd"=w1117, "type"=w1118) -> ("success"=w1119:bool)  [unwired: 8 in, 1 out]
                        n399 = case shown="真" w1119 {
                          tunnel: [w1120 w1122] -> w1116
                          frame False {
                            n400 = call "sub-Language-get str-const.vi"("sid"=u32 260) -> ("str"=w1120:string)
                          }
                          frame True {
                            n401 = call "sub-Language-get str-const.vi"("sid"=u32 259) -> ("str"=w1122:string)
                          }
                        }
                      }
                    }
                  }
                }
                n402 = global write "_USB_CAN_GLOBAL_.vi" "open"(FALSE ("open")) -> ()
                n403 = call "Global_Application Path.vi"("Use ExeFilePath"=FALSE) -> ("程序路径"=w1084:path)
                n404 = Build Path(base path=w1084, name or relative path="BR Detect.exe " ("command line")) -> (appended path=w1082:path)
                n405 = Path To String(path=w1082) -> (string=w1081:string)
                n406 = call <vilib>:"System Exec.vi"("wait until completion? (T)"=FALSE, "command line"=w1081) -> ("error out"=w1079:errorcluster)  [unwired: 6 in, 3 out]
                n407 = case shown="错误" w1079 {
                  tunnel: w1078 -> [w1096 _]
                  frame No Error {
                    n408 = call "sub-Language-get str-const.vi"("sid"=u32 256) -> ("str"=w1093:string)
                    n409 = Empty String/Path?(string/path=w1096) -> (empty?=w1095:bool)
                    n410 = case shown="假" w1095 {
                      tunnel: w1096 -> [w1098 _]
                      tunnel: w1093 -> [w1097 _]
                      frame False {
                        n411 = call "TimeLmtDialog.vi"("Infoin"=w1098, "title"=w1097) -> ()  [unwired: 10 in]
                      }
                      frame True {
                      }
                    }
                  }
                  frame Error {
                    n412 = call "sub-Language-get str-const.vi"("sid"=u32 262) -> ("str"=w1099:string)
                    n413 = call "sub-Language-get str-const.vi"("sid"=u32 261) -> ("str"=w1101:string)
                    n414 = call "TimeLmtDialog.vi"("Infoin"=w1099, "title"=w1101) -> ()  [unwired: 10 in]
                  }
                }
                n415 = property class="VI"("Front Panel.Title"=w1088) -> ()  [unwired: 2 in, 2 out]
              }
              frame "m000D" {
                w1133 = FALSE
                n416 = case shown="真" w1137 {
                  tunnel: w1136 -> [_ w1151]
                  tunnel: [_ w1149] -> w1125
                  frame False {
                  }
                  frame True {
                    n417 = local read "DevIndex"() -> (w1150:u32)
                    n418 = stacked-sequence {
                      tunnel: w1151 -> [w1153 w1165]
                      tunnel: w1150 -> [w1152 w1164]
                      tunnel: [_ w1163] -> w1149
                      frame #0 {
                        n419 = Equal?(x=w1153, y=u16 4) -> (x = y?=w1157:bool)
                        n420 = Select(t=2, s=w1157, f=1) -> (s? t:f=w1154:i32)
                        n421 = for {
                          N: w1154 -> [_]
                          tunnel: w1153 -> [w1161]
                          tunnel: w1152 -> [w1160]
                          i -> [w1159]
                          n422 = call "ResetCAN.vi"("CANInd"=w1159, "DeciceInd"=w1160, "DeviceType"=w1161) -> ()  [unwired: 7 in, 2 out]
                        }
                      }
                      frame #1 {
                        n423 = call "CloseDevice.vi"("DeviceInd"=w1164, "type"=w1165) -> ("success"=w1162:bool)  [unwired: 8 in, 1 out]
                        n424 = case shown="真" w1162 {
                          tunnel: [w1166 w1168] -> w1163
                          frame False {
                            n425 = call "sub-Language-get str-const.vi"("sid"=u32 260) -> ("str"=w1166:string)
                          }
                          frame True {
                            n426 = call "sub-Language-get str-const.vi"("sid"=u32 259) -> ("str"=w1168:string)
                          }
                        }
                      }
                    }
                  }
                }
                n427 = global write "_USB_CAN_GLOBAL_.vi" "open"(FALSE ("open")) -> ()
                n428 = call "Global_Application Path.vi"("Use ExeFilePath"=FALSE) -> ("程序路径"=w1130:path)
                n429 = Build Path(base path=w1130, name or relative path="CANBridgeConfig.exe " ("command line")) -> (appended path=w1128:path)
                n430 = Path To String(path=w1128) -> (string=w1127:string)
                n431 = call <vilib>:"System Exec.vi"("wait until completion? (T)"=FALSE, "command line"=w1127) -> ("error out"=w1124:errorcluster)  [unwired: 6 in, 3 out]
                n432 = case shown="错误" w1124 {
                  tunnel: w1125 -> [w1142 _]
                  frame No Error {
                    n433 = call "sub-Language-get str-const.vi"("sid"=u32 256) -> ("str"=w1139:string)
                    n434 = Empty String/Path?(string/path=w1142) -> (empty?=w1141:bool)
                    n435 = case shown="假" w1141 {
                      tunnel: w1142 -> [w1144 _]
                      tunnel: w1139 -> [w1143 _]
                      frame False {
                        n436 = call "TimeLmtDialog.vi"("Infoin"=w1144, "title"=w1143) -> ()  [unwired: 10 in]
                      }
                      frame True {
                      }
                    }
                  }
                  frame Error {
                    n437 = call "sub-Language-get str-const.vi"("sid"=u32 261) -> ("str"=w1147:string)
                    n438 = call "sub-Language-get str-const.vi"("sid"=u32 262) -> ("str"=w1145:string)
                    n439 = call "TimeLmtDialog.vi"("Infoin"=w1145, "title"=w1147) -> ()  [unwired: 10 in]
                  }
                }
                n440 = property class="VI"("Front Panel.Title"=w1134) -> ()  [unwired: 2 in, 2 out]
              }
              frame "m000E" {
                w1179 = FALSE
                n441 = case shown="真" w1183 {
                  tunnel: w1182 -> [_ w1197]
                  tunnel: [_ w1195] -> w1170
                  frame False {
                  }
                  frame True {
                    n442 = local read "DevIndex"() -> (w1196:u32)
                    n443 = stacked-sequence {
                      tunnel: w1197 -> [w1199 w1211]
                      tunnel: w1196 -> [w1198 w1210]
                      tunnel: [_ w1208] -> w1195
                      frame #0 {
                        n444 = Equal?(x=w1199, y=u16 4) -> (x = y?=w1203:bool)
                        n445 = Select(t=2, s=w1203, f=1) -> (s? t:f=w1200:i32)
                        n446 = for {
                          N: w1200 -> [_]
                          tunnel: w1199 -> [w1207]
                          tunnel: w1198 -> [w1206]
                          i -> [w1205]
                          n447 = call "ResetCAN.vi"("CANInd"=w1205, "DeciceInd"=w1206, "DeviceType"=w1207) -> ()  [unwired: 7 in, 2 out]
                        }
                      }
                      frame #1 {
                        n448 = call "CloseDevice.vi"("DeviceInd"=w1210, "type"=w1211) -> ("success"=w1209:bool)  [unwired: 8 in, 1 out]
                        n449 = case shown="真" w1209 {
                          tunnel: [w1212 w1214] -> w1208
                          frame False {
                            n450 = call "sub-Language-get str-const.vi"("sid"=u32 260) -> ("str"=w1212:string)
                          }
                          frame True {
                            n451 = call "sub-Language-get str-const.vi"("sid"=u32 259) -> ("str"=w1214:string)
                          }
                        }
                      }
                    }
                  }
                }
                n452 = global write "_USB_CAN_GLOBAL_.vi" "open"(FALSE ("open")) -> ()
                n453 = call "Global_Application Path.vi"("Use ExeFilePath"=FALSE) -> ("程序路径"=w1176:path)
                n454 = Build Path(base path=w1176, name or relative path="USBCAN Test.exe " ("command line")) -> (appended path=w1174:path)
                n455 = Path To String(path=w1174) -> (string=w1172:string)
                n456 = call <vilib>:"System Exec.vi"("wait until completion? (T)"=FALSE, "command line"=w1172) -> ("error out"=w1171:errorcluster)  [unwired: 6 in, 3 out]
                n457 = case shown="错误" w1171 {
                  tunnel: w1170 -> [w1188 _]
                  frame No Error {
                    n458 = call "sub-Language-get str-const.vi"("sid"=u32 256) -> ("str"=w1185:string)
                    n459 = Empty String/Path?(string/path=w1188) -> (empty?=w1187:bool)
                    n460 = case shown="假" w1187 {
                      tunnel: w1188 -> [w1190 _]
                      tunnel: w1185 -> [w1189 _]
                      frame False {
                        n461 = call "TimeLmtDialog.vi"("Infoin"=w1190, "title"=w1189) -> ()  [unwired: 10 in]
                      }
                      frame True {
                      }
                    }
                  }
                  frame Error {
                    n462 = call "sub-Language-get str-const.vi"("sid"=u32 262) -> ("str"=w1191:string)
                    n463 = call "sub-Language-get str-const.vi"("sid"=u32 261) -> ("str"=w1193:string)
                    n464 = call "TimeLmtDialog.vi"("Infoin"=w1191, "title"=w1193) -> ()  [unwired: 10 in]
                  }
                }
                n465 = property class="VI"("Front Panel.Title"=w1180) -> ()  [unwired: 2 in, 2 out]
              }
              frame "m000B" {
                n466 = global read "_USB_CAN_GLOBAL_.vi" "open"() -> (w1218:bool)
                n467 = case shown="假" w1218 {
                  tunnel: w1217 -> [_ w1227]
                  frame False {
                    n468 = call "sub-Language-get str-const.vi"("sid"=u32 263) -> ("str"=w1222:string)
                    n469 = call "sub-Language-get str-const.vi"("sid"=u32 256) -> ("str"=w1224:string)
                    n470 = call "TimeLmtDialog.vi"("Infoin"=w1222, "title"=w1224) -> ()  [unwired: 10 in]
                  }
                  frame True {
                    n471 = local read "DevIndex"() -> (w1226:u32)
                    n472 = call "CanStatusShow.vi"("DevIndex"=w1226, "DevType"=w1227) -> ()  [unwired: 10 in]
                  }
                }
              }
              frame "m000F" {
                n473 = global read "_USB_CAN_GLOBAL_.vi" "open"() -> (w1230:bool)
                n474 = case shown="真" w1230 {
                  selector: w1230 -> [_ w1246]
                  tunnel: w1235 -> [w1241 w1245]
                  tunnel: [w1241 w1244] -> w1234
                  tunnel: w1233 -> [_ w1247]
                  tunnel: w1229 -> [_ w1243]
                  tunnel: w1228 -> [_ w1242]
                  frame False {
                    n475 = call "sub-Language-get str-const.vi"("sid"=u32 263) -> ("str"=w1237:string)
                    n476 = call "sub-Language-get str-const.vi"("sid"=u32 256) -> ("str"=w1239:string)
                    n477 = call "TimeLmtDialog.vi"("Infoin"=w1237, "title"=w1239) -> ()  [unwired: 10 in]
                  }
                  frame True {
                    n478 = stacked-sequence {
                      tunnel: w1247 -> [_ w1264 _]
                      tunnel: w1246 -> [_ w1263 _]
                      tunnel: w1245 -> [_ w1260 _]
                      tunnel: [_ w1259 _] -> w1244
                      tunnel: w1243 -> [_ _ w1275]
                      tunnel: w1242 -> [w1251 _ _]
                      frame #0 {
                        w1249 = FALSE
                        n479 = invoke class="VI" method="Ctrl Val.Set"(reference=w1251, "Control Name"="Enable" ("控件名"), "Value"=w1249) -> ()  [unwired: 2 in, 5 out]
                        n480 = Open VI Reference(vi path=path "DeviceOP/ReciveThread.vi" ("VI路径")) -> (vi reference=w1252:refnum<vi>, error out=w1253:errorcluster)  [unwired: 5 in]
                        n481 = invoke class="VI" method="Ctrl Val.Set"(reference=w1252, error in=w1253, "Control Name"="Enable1" ("控件名"), "Value"=w1249) -> (reference out=w1256:refnum<vi>, error out=w1257:errorcluster)  [unwired: 1 in, 3 out]
                        n482 = Not(x=w1249) -> (.not. x?=w1248:bool)
                        n483 = invoke class="VI" method="Ctrl Val.Set"(reference=w1256, error in=w1257, "Control Name"="Enable2" ("控件名"), "Value"=w1249) -> ()  [unwired: 1 in, 5 out]
                        n484 = property on="send stop" class="Bool (严格)"("Val(Sgnl)"=w1248) -> ()  [unwired: 2 in, 2 out]
                      }
                      frame #1 {
                        n485 = local read "DevIndex"() -> (w1265:u32)
                        n486 = call "CAN-SET.vi"("DevIndex"=w1265, "open?"=w1263, "type"=w1264) -> ("success"=w1262:bool, "Param out"=w1261:T5[])  [unwired: 7 in]
                        n487 = Select(t=w1261, s=w1262, f=w1260) -> (s? t:f=w1259:T5[])
                      }
                      frame #2 {
                        n488 = Unbundle By Name(w1275) -> ("RcvE1"=w1274:bool, "RcvE2"=w1273:bool)
                        n489 = Open VI Reference(vi path=path "DeviceOP/ReciveThread.vi" ("VI路径")) -> (vi reference=w1266:refnum<vi>, error out=w1267:errorcluster)  [unwired: 5 in]
                        n490 = invoke class="VI" method="Ctrl Val.Set"(reference=w1266, error in=w1267, "Control Name"="Enable1" ("控件名"), "Value"=w1274) -> (reference out=w1270:refnum<vi>, error out=w1271:errorcluster)  [unwired: 1 in, 3 out]
                        n491 = invoke class="VI" method="Ctrl Val.Set"(reference=w1270, error in=w1271, "Control Name"="Enable2" ("控件名"), "Value"=w1273) -> ()  [unwired: 1 in, 5 out]
                      }
                    }
                  }
                }
              }
              frame "m0010" {
                n492 = Unbundle By Name(w1292) -> ("scantime"=w1294:u16)
                n493 = Open VI Reference(vi path=path "DeviceOP/ReciveThread.vi" ("VI路径")) -> (vi reference=w1288:refnum<vi>, error out=w1287:errorcluster)  [unwired: 5 in]
                n494 = call "Scan time Input.vi"("In"=w1294) -> ("out"=w1286:u32)  [unwired: 10 in]
                n495 = Bundle By Name(cluster=w1292, "scantime"=w1286) -> (w1291:T2)
                n496 = Get Menu Item Info(7:w1283, 11:w1285) -> (2:w1281:string, 3:w1284:refnum<k9>)  [unwired: 1 in, 5 out]
                n497 = invoke class="VI" method="Ctrl Val.Set"(reference=w1288, error in=w1287, "Control Name"="Scan time" ("控件名"), "Value"=w1286) -> ()  [unwired: 1 in, 5 out]
                n498 = call "sub-Get menu shortkey str.vi"("menu desc"=w1281) -> ("short key str"=w1277:string, "menu desc split"=w1280:string)  [unwired: 9 in]
                n499 = Match Pattern(string=w1280, regular expression="([0-9]+ms)" ("正则表达式")) -> (before substring=w1279:string)  [unwired: 1 in, 3 out]
                n500 = Concatenate Strings(w1279, "(%dms)" ("格式字符串"), w1277) -> (w1276:string)
                n501 = Format Into String(format string=w1276, w1286) -> (resulting string=w1293:string)  [unwired: 2 in, 1 out]
                n502 = Set Menu Item Info(7:w1283, 10:w1293, 11:w1284) -> ()  [unwired: 4 in, 2 out]
              }
              frame "m0011" {
                n503 = Unbundle By Name(w1318) -> ("RcvLen"=w1316:i16)
                n504 = Open VI Reference(vi path=path "DeviceOP/ReciveThread.vi" ("VI路径")) -> (vi reference=w1312:refnum<vi>, error out=w1311:errorcluster)  [unwired: 5 in]
                n505 = call "Scan time Input.vi"("In"=w1316) -> ("out"=w1310:u32)  [unwired: 10 in]
                n506 = Bundle By Name(cluster=w1318, "RcvLen"=w1310) -> (w1317:T2)
                n507 = Get Menu Item Info(7:w1307, 11:w1308) -> (2:w1305:string, 3:w1306:refnum<k9>)  [unwired: 1 in, 5 out]
                n508 = call "sub-Get menu shortkey str.vi"("menu desc"=w1305) -> ("short key str"=w1301:string, "menu desc split"=w1304:string)  [unwired: 9 in]
                n509 = invoke class="VI" method="Ctrl Val.Set"(reference=w1312, error in=w1311, "Control Name"="RcvLen" ("控件名"), "Value"=w1310) -> ()  [unwired: 1 in, 5 out]
                n510 = Match Pattern(string=w1304, regular expression="([0-9]+)" ("正则表达式")) -> (before substring=w1303:string)  [unwired: 1 in, 3 out]
                n511 = Concatenate Strings(w1303, "(%d)" ("格式字符串"), w1301) -> (w1300:string)
                n512 = Format Into String(format string=w1300, w1310) -> (resulting string=w1315:string)  [unwired: 2 in, 1 out]
                n513 = Set Menu Item Info(7:w1307, 10:w1315, 11:w1306) -> ()  [unwired: 4 in, 2 out]
              }
              frame "m0012" {
                n514 = Unbundle By Name(w1340) -> ("BuffLen"=w1338:u16)
                n515 = call "Scan time Input.vi"("In"=w1338) -> ("out"=w1335:u32)  [unwired: 10 in]
                n516 = Bundle By Name(cluster=w1340, "BuffLen"=w1335) -> (w1339:T2)
                n517 = Get Menu Item Info(7:w1330, 11:w1332) -> (2:w1327:string, 3:w1331:refnum<k9>)  [unwired: 1 in, 5 out]
                n518 = call "sub-Get menu shortkey str.vi"("menu desc"=w1327) -> ("short key str"=w1324:string, "menu desc split"=w1326:string)  [unwired: 9 in]
                n519 = invoke class="VI" method="Ctrl Val.Set"(reference=w1334, "Control Name"="BuffLen" ("控件名"), "Value"=w1335) -> ()  [unwired: 2 in, 5 out]
                n520 = Match Pattern(string=w1326, regular expression="([0-9]+)" ("正则表达式")) -> (before substring=w1325:string)  [unwired: 1 in, 3 out]
                n521 = Concatenate Strings(w1325, "(%d)" ("格式字符串"), w1324) -> (w1328:string)
                n522 = Format Into String(format string=w1328, w1335) -> (resulting string=w1337:string)  [unwired: 2 in, 1 out]
                n523 = Set Menu Item Info(7:w1330, 10:w1337, 11:w1331) -> ()  [unwired: 4 in, 2 out]
              }
              frame "m0015" {
                # "USB掉线重启..."
                # "USB掉线重连模式"
                n524 = Unbundle By Name(w1348) -> ("autoconn"=w1349:bool)
                n525 = Not(x=w1349) -> (.not. x?=w1346:bool)
                n526 = Set Menu Item Info(6:w1346, 7:w1351, 11:w1350) -> ()  [unwired: 4 in, 2 out]
                n527 = case shown="假" w1346 {
                  frame False {
                    n528 = property class="VI"() -> ("Front Panel.Title"=w1362:string)  [unwired: 2 in, 2 out]
                    n529 = call "sub-Language-get str-const.vi"("sid"=u32 264) -> ("str"=w1359:string)
                    n530 = call "sub-Language-get str-const.vi"("sid"=u32 265) -> ("str"=w1357:string)
                    n531 = Search and Replace String(input string=w1362, search string=w1359, replace string=w1357) -> (result string=w1361:string)  [unwired: 5 in, 3 out]
                    n532 = property class="VI"("Front Panel.Title"=w1361) -> ()  [unwired: 2 in, 2 out]
                  }
                  frame True {
                    n533 = call "important information-autoConn1.vi"() -> ()  [unwired: 12 in]
                  }
                }
                n534 = Bundle By Name(cluster=w1348, "autoconn"=w1346) -> (w1347:T2)
              }
              frame "m0036" {
                n535 = Get Menu Item Info(7:w1373, 11:w1374) -> (3:w1376:refnum<k9>, 4:w1375:bool)  [unwired: 1 in, 5 out]
                n536 = Not(x=w1375) -> (.not. x?=w1366:bool)
                n537 = Set Menu Item Info(6:w1366, 7:w1373, 11:w1376) -> ()  [unwired: 4 in, 2 out]
                n538 = invoke class="VI" method="Ctrl Val.Set"(reference=w1372, "Control Name"="check1" ("控件名"), "Value"=w1366) -> ()  [unwired: 2 in, 5 out]
                n539 = Select(t=T4."Enabled" ("禁用"), s=w1366, f=T4."Disabled and Grayed Out" ("禁用")) -> (s? t:f=w1363:T4)
                n540 = Bundle By Name(cluster=w1369, "chk1"=w1366) -> (w1370:T2)
                n541 = property on="errcnt1" class="DigNum (严格)"("DisabledEnum"=w1363) -> ()  [unwired: 2 in, 2 out]
              }
              frame "m0037" {
                n542 = Get Menu Item Info(7:w1394, 11:w1395) -> (3:w1397:refnum<k9>, 4:w1396:bool)  [unwired: 1 in, 5 out]
                n543 = Not(x=w1396) -> (.not. x?=w1381:bool)
                n544 = Set Menu Item Info(6:w1381, 7:w1394, 11:w1397) -> ()  [unwired: 4 in, 2 out]
                n545 = Unbundle By Name(w1385) -> ("type"=w1384:u16)
                n546 = Equal?(x=u16 4, y=w1384) -> (x = y?=w1382:bool)
                n547 = And(x=w1382, y=w1381) -> (x .and. y?=w1380:bool)
                n548 = Bundle By Name(cluster=w1385, "chk2"=w1381) -> (w1391:T2)
                n549 = invoke class="VI" method="Ctrl Val.Set"(reference=w1393, "Control Name"="check2" ("控件名"), "Value"=w1380) -> ()  [unwired: 2 in, 5 out]
                n550 = Select(t=T4."Enabled" ("禁用"), s=w1380, f=T4."Disabled and Grayed Out" ("禁用")) -> (s? t:f=w1386:T4)
                n551 = property on="errcnt2" class="DigNum (严格)"("DisabledEnum"=w1386) -> ()  [unwired: 2 in, 2 out]
              }
              frame "m0026" {
                n552 = Get Menu Item Info(7:w1410, 11:w1411) -> (3:w1413:refnum<k9>, 4:w1412:bool)  [unwired: 1 in, 5 out]
                n553 = Not(x=w1412) -> (.not. x?=w1401:bool)
                n554 = Set Menu Item Info(6:w1401, 7:w1410, 11:w1413) -> ()  [unwired: 4 in, 2 out]
                n555 = Open VI Reference(vi path=path "DeviceOP/ReciveThread.vi" ("VI路径")) -> (vi reference=w1404:refnum<vi>, error out=w1402:errorcluster)  [unwired: 5 in]
                n556 = invoke class="VI" method="Ctrl Val.Set"(reference=w1404, error in=w1402, "Control Name"="Enable1" ("控件名"), "Value"=w1401) -> ()  [unwired: 1 in, 5 out]
                n557 = Bundle By Name(cluster=w1408, "RcvE1"=w1401) -> (w1409:T2)
              }
              frame "m0027" {
                n558 = Get Menu Item Info(7:w1430, 11:w1431) -> (3:w1433:refnum<k9>, 4:w1432:bool)  [unwired: 1 in, 5 out]
                n559 = Not(x=w1432) -> (.not. x?=w1418:bool)
                n560 = Set Menu Item Info(6:w1418, 7:w1430, 11:w1433) -> ()  [unwired: 4 in, 2 out]
                n561 = Unbundle By Name(w1419) -> ("type"=w1422:u16)
                n562 = Open VI Reference(vi path=path "DeviceOP/ReciveThread.vi" ("VI路径")) -> (vi reference=w1425:refnum<vi>, error out=w1423:errorcluster)  [unwired: 5 in]
                n563 = Equal?(x=u16 4, y=w1422) -> (x = y?=w1420:bool)
                n564 = And(x=w1420, y=w1418) -> (x .and. y?=w1417:bool)
                n565 = invoke class="VI" method="Ctrl Val.Set"(reference=w1425, error in=w1423, "Control Name"="Enable2" ("控件名"), "Value"=w1417) -> ()  [unwired: 1 in, 5 out]
                n566 = Bundle By Name(cluster=w1419, "RcvE2"=w1417) -> (w1429:T2)
              }
              frame "m0016" {
                # "恢复出厂设置（软件参数重置）"
                n567 = call "sub-Language-get str-const.vi"("sid"=u32 266) -> ("str"=w1437:string)
                n568 = call "sub-Language-get str-const.vi"("sid"=u32 267) -> ("str"=w1441:string)
                n569 = call "sub-Language-get str-const.vi"("sid"=u32 268) -> ("str"=w1439:string)
                n570 = Two Button Dialog(message=w1437, 1:w1439, 2:w1441) -> (T button?=w1443:bool)
                n571 = case shown="真" w1443 {
                  tunnel: w1444 -> [_ w1450]
                  frame False {
                  }
                  frame True {
                    n572 = stacked-sequence {
                      tunnel: w1450 -> [_ _ w1476 _ _]
                      frame #0 {
                        n573 = call "Global_Application Path.vi"() -> ("程序路径"=w1457:path)  [unwired: 1 in]
                        n574 = call "Global_Application Path.vi"() -> ("程序路径"=w1452:path)  [unwired: 1 in]
                        n575 = Build Path(base path=w1457, name or relative path="usb_can.ini" ("名称或相对路径")) -> (appended path=w1456:path)
                        n576 = Build Path(base path=w1452, name or relative path="USB_CAN Debug.log" ("名称或相对路径")) -> (appended path=w1453:path)
                        n577 = Delete(path (use dialog)=w1456) -> (error out=w1455:errorcluster)  [unwired: 4 in, 2 out]
                        n578 = Delete(path (use dialog)=w1453) -> (error out=w1454:errorcluster)  [unwired: 4 in, 2 out]
                        n579 = call <vilib>:"Clear Errors.vi"("error in (no error)"=w1455) -> ()  [unwired: 6 in, 1 out]
                        n580 = call <vilib>:"Clear Errors.vi"("error in (no error)"=w1454) -> ()  [unwired: 6 in, 1 out]
                      }
                      frame #1 {
                        n581 = property class="VI"() -> ("Name"=w1465:string)  [unwired: 2 in, 2 out]
                        n582 = call "Global_Application Path.vi"() -> ("程序路径"=w1462:path)  [unwired: 1 in]
                        n583 = String To Byte Array(string=w1465) -> (unsigned byte array=w1464:u8[])
                        n584 = for {
                          N: 4 -> [_]
                          tunnel: w1464 -> [w1474] mode=indexing
                          shift-right: [w1471] -> w1466
                          shift-left: "" -> [w1472]
                          n585 = Format Into String(format string="%02x" ("格式字符串"), initial string=w1472, w1474) -> (resulting string=w1471:string)  [unwired: 1 in, 1 out]
                        }
                        n586 = String Subset(string=w1466, length (rest)=16 ("长度（剩余）")) -> (substring=w1468:string)  [unwired: 1 in]
                        n587 = Concatenate Strings(w1468, ".uis" ("字符串")) -> (w1461:string)
                        n588 = Build Path(base path=w1462, name or relative path=w1461) -> (appended path=w1460:path)
                        n589 = Delete(path (use dialog)=w1460) -> (error out=w1459:errorcluster)  [unwired: 4 in, 2 out]
                        n590 = call <vilib>:"Clear Errors.vi"("error in (no error)"=w1459) -> ()  [unwired: 6 in, 1 out]
                      }
                      frame #2 {
                        n591 = local read "DevIndex"() -> (w1475:u32)
                        n592 = call "CloseDevice.vi"("DeviceInd"=w1475, "type"=w1476) -> ()  [unwired: 8 in, 2 out]
                      }
                      frame #3 {
                        n593 = call "Global_Application Path.vi"() -> ("程序路径"=w1483:path)  [unwired: 1 in]
                        n594 = call "Global_Application Path.vi"("Use ExeFilePath"=TRUE) -> ("程序路径"=w1482:path)
                        n595 = Path To String(path=w1482) -> (string=w1480:string)
                        n596 = Concatenate Strings("reboot.exe -- run \"" ("command line"), w1480, "\" w:4000 \"t:USB_CAN Tool -- Reboot\"" ("字符串")) -> (w1479:string)
                        n597 = call <vilib>:"System Exec.vi"("wait until completion? (T)"=FALSE, "working directory"=w1483, "command line"=w1479) -> ("error out"=w1484:errorcluster)  [unwired: 5 in, 3 out]
                        n598 = call <vilib>:"Clear Errors.vi"("error in (no error)"=w1484) -> ()  [unwired: 6 in, 1 out]
                      }
                      frame #4 {
                        n599 = control-ref of="本VI"() -> (w1486:refnum<vi>)
                        n600 = call "Exit.vi"("VI引用"=w1486) -> ()  [unwired: 10 in, 1 out]
                      }
                    }
                  }
                }
              }
              frame "m0017" {
                n601 = Equal?(x=w1487, y=u16 4) -> (x = y?=w1491:bool)
                n602 = Select(t=2, s=w1491, f=1) -> (s? t:f=w1488:i32)
                n603 = for {
                  N: w1488 -> [_]
                  tunnel: w1487 -> [w1506]
                  tunnel: [w1504] -> w1496 mode=indexing
                  tunnel: [w1503] -> w1493 mode=indexing
                  i -> [w1501]
                  w1502 = u32 15 items=["REFTYPE_MODE"=0, "REFTYPE_FILTER"=1, "REFTYPE_ACR0"=2, "REFTYPE_AMR0"=6, "REFTYPE_kCANBAUD"=10, "REFTYPE_CANRX_EN"=13, "REFTYPE_UARTBAUD"=14, "REFTYPE_ALL"=15] ("RefType")
                  n604 = local read "DevIndex"() -> (w1505:u32)
                  n605 = call "GetReference2.vi"("DeviceType"=w1506, "DeviceInd"=w1505, "CANInd"=w1501, "RefType"=w1502) -> ("Success"=w1504:bool, "Param"=w1503:T5)  [unwired: 9 in, 1 out]
                }
                n606 = And Array Elements(Boolean array=w1496) -> (logical AND=w1495:bool)
                n607 = case shown="真" w1495 {
                  tunnel: w1493 -> [_ w1512]
                  tunnel: w1487 -> [_ w1511]
                  frame False {
                    n608 = call "sub-Language-get str-const.vi"("sid"=u32 269) -> ("str"=w1507:string)
                    n609 = call "sub-Language-get str-const.vi"("sid"=u32 256) -> ("str"=w1509:string)
                    n610 = call "TimeLmtDialog.vi"("Infoin"=w1507, "title"=w1509) -> ()  [unwired: 10 in]
                  }
                  frame True {
                    n611 = call "CAN_ParamShow.vi"("DevType"=w1511, "param"=w1512) -> ()  [unwired: 10 in]
                  }
                }
              }
              frame "m0018" {
                n612 = case shown="真" w1516 {
                  tunnel: w1515 -> [_ w1526]
                  frame False {
                    n613 = call "sub-Language-get str-const.vi"("sid"=u32 270) -> ("str"=w1519:string)
                    n614 = call "sub-Language-get str-const.vi"("sid"=u32 256) -> ("str"=w1521:string)
                    n615 = call "TimeLmtDialog.vi"("Infoin"=w1519, "title"=w1521) -> ()  [unwired: 10 in]
                  }
                  frame True {
                    n616 = local read "DevIndex"() -> (w1525:u32)
                    n617 = call "ReadBoardInfo.vi"("DeviceInd"=w1525, "DeviceType"=w1526) -> ("VCI_BOARD_INFO"=w1523:T7, "success"=w1524:bool)  [unwired: 8 in]
                    n618 = case shown="真" w1524 {
                      tunnel: w1523 -> [_ w1531]
                      frame False {
                        n619 = call "sub-Language-get str-const.vi"("sid"=u32 256) -> ("str"=w1529:string)
                        n620 = call "sub-Language-get str-const.vi"("sid"=u32 269) -> ("str"=w1527:string)
                        n621 = call "TimeLmtDialog.vi"("Infoin"=w1527, "title"=w1529) -> ()  [unwired: 10 in]
                      }
                      frame True {
                        n622 = call "_USB_CAN_BOARD_INFO_.vi"("VCI_BOARD_INFO"=w1531) -> ()  [unwired: 11 in]
                      }
                    }
                  }
                }
              }
              frame "m0019" {
                # "12"
                n623 = Get Menu Item Info(7:w1543, 11:w1545) -> (3:w1544:refnum<k9>, 4:w1542:bool)  [unwired: 1 in, 5 out]
                n624 = Not(x=w1542) -> (.not. x?=w1533:bool)
                n625 = Set Menu Item Info(6:w1533, 7:w1543, 11:w1544) -> (3:w1534:refnum<k9>)  [unwired: 4 in, 1 out]
                n626 = invoke class="VI" method="Ctrl Val.Set"(reference=w1541, "Control Name"="highspd" ("控件名"), "Value"=w1533) -> ()  [unwired: 2 in, 5 out]
                n627 = Not(x=w1533) -> (.not. x?=w1532:bool)
                n628 = Set Menu Item Info(7:"m001A" ("项标识符"), 9:w1532, 11:w1534) -> ()  [unwired: 4 in, 2 out]
                n629 = Bundle By Name(cluster=w1539, "highspd"=w1533) -> (w1538:T2)
              }
              frame "m001A" {
                n630 = Get Menu Item Info(7:w1557, 11:w1559) -> (3:w1558:refnum<k9>, 4:w1556:bool)  [unwired: 1 in, 5 out]
                n631 = Not(x=w1556) -> (.not. x?=w1553:bool)
                n632 = Set Menu Item Info(6:w1553, 7:w1557, 11:w1558) -> ()  [unwired: 4 in, 2 out]
                n633 = invoke class="VI" method="Ctrl Val.Set"(reference=w1555, "Control Name"="disp" ("控件名"), "Value"=w1553) -> ()  [unwired: 2 in, 5 out]
                n634 = Bundle By Name(cluster=w1552, "disp"=w1553) -> (w1551:T2)
              }
              frame "m001B" {
                n635 = Get Menu Item Info(7:w1569, 11:w1571) -> (3:w1570:refnum<k9>, 4:w1568:bool)  [unwired: 1 in, 5 out]
                n636 = Not(x=w1568) -> (.not. x?=w1563:bool)
                n637 = Set Menu Item Info(6:w1563, 7:w1569, 11:w1570) -> ()  [unwired: 4 in, 2 out]
                n638 = global write "_USB_CAN_GLOBAL_.vi" "Disp-HL"(w1563) -> ()
                n639 = Bundle By Name(cluster=w1567, "hl"=w1563) -> (w1566:T2)
              }
              frame "m0030" {
                n640 = Get Menu Item Info(7:w1592, 11:w1593) -> (3:w1587:refnum<k9>, 4:w1585:bool)  [unwired: 1 in, 5 out]
                n641 = Set Menu Item Info(6:w1585, 7:"m0031" ("项标识符"), 11:w1587) -> (3:w1584:refnum<k9>)  [unwired: 4 in, 1 out]
                n642 = Not(x=w1585) -> (.not. x?=w1583:bool)
                n643 = Set Menu Item Info(6:w1583, 7:w1592, 11:w1584) -> ()  [unwired: 4 in, 2 out]
                n644 = Select(t=enum16{"原始值", "实际值"}."原始值" ("TSFormat"), s=w1583, f=enum16{"原始值", "实际值"}."实际值" ("TSFormat")) -> (s? t:f=w1579:enum16{"原始值", "实际值"})
                n645 = invoke class="VI" method="Ctrl Val.Set"(reference=w1580, "Control Name"="TSFormat" ("控件名"), "Value"=w1579) -> (reference out=w1575:refnum<vi>)  [unwired: 2 in, 4 out]
                n646 = Bundle By Name(cluster=w1591, "TSFormat"=w1579) -> (w1590:T2)
                n647 = invoke class="VI" method="Ctrl Val.Set"(reference=w1575, "Control Name"="ForceUpt" ("控件名"), "Value"=TRUE) -> ()  [unwired: 2 in, 5 out]
              }
              frame "m0031" {
                n648 = Get Menu Item Info(7:w1614, 11:w1615) -> (3:w1609:refnum<k9>, 4:w1607:bool)  [unwired: 1 in, 5 out]
                n649 = Set Menu Item Info(6:w1607, 7:"m0030" ("项标识符"), 11:w1609) -> (3:w1606:refnum<k9>)  [unwired: 4 in, 1 out]
                n650 = Not(x=w1607) -> (.not. x?=w1605:bool)
                n651 = Set Menu Item Info(6:w1605, 7:w1614, 11:w1606) -> ()  [unwired: 4 in, 2 out]
                n652 = Select(t=enum16{"原始值", "实际值"}."实际值" ("TSFormat"), s=w1605, f=enum16{"原始值", "实际值"}."原始值" ("TSFormat")) -> (s? t:f=w1601:enum16{"原始值", "实际值"})
                n653 = invoke class="VI" method="Ctrl Val.Set"(reference=w1602, "Control Name"="TSFormat" ("控件名"), "Value"=w1601) -> (reference out=w1597:refnum<vi>)  [unwired: 2 in, 4 out]
                n654 = Bundle By Name(cluster=w1613, "TSFormat"=w1601) -> (w1612:T2)
                n655 = invoke class="VI" method="Ctrl Val.Set"(reference=w1597, "Control Name"="ForceUpt" ("控件名"), "Value"=TRUE) -> ()  [unwired: 2 in, 5 out]
              }
              frame "m001C" {
                n656 = Get Menu Item Info(7:w1630, 11:w1632) -> (3:w1631:refnum<k9>, 4:w1629:bool)  [unwired: 1 in, 5 out]
                n657 = Not(x=w1629) -> (.not. x?=w1625:bool)
                n658 = Set Menu Item Info(6:w1625, 7:w1630, 11:w1631) -> ()  [unwired: 4 in, 2 out]
                n659 = invoke class="VI" method="Ctrl Val.Set"(reference=w1628, "Control Name"="ID合并" ("控件名"), "Value"=w1625) -> (reference out=w1621:refnum<vi>)  [unwired: 2 in, 4 out]
                n660 = Bundle By Name(cluster=w1626, "ID合并"=w1625) -> (w1624:T2)
                n661 = invoke class="VI" method="Ctrl Val.Set"(reference=w1621, "Control Name"="ForceUpt" ("控件名"), "Value"=TRUE) -> ()  [unwired: 2 in, 5 out]
              }
              frame "m0028", "m0029", "m002A", "m002B" {
                n662 = Get Menu Item Info(7:"m001D" ("项标识符"), 11:w1642) -> (2:w1640:string)  [unwired: 1 in, 6 out]
                n663 = case shown="\"m0029\"" w1653 {
                  tunnel: [TRUE FALSE FALSE FALSE] -> w1657
                  tunnel: [FALSE TRUE FALSE FALSE] -> w1656
                  tunnel: [FALSE FALSE TRUE FALSE] -> w1655
                  tunnel: [FALSE FALSE FALSE TRUE] -> w1654
                  tunnel: [enum16{"hex", "dec", "oct", "bin"}."hex" ("format") enum16{"hex", "dec", "oct", "bin"}."dec" ("format") enum16{"hex", "dec", "oct", "bin"}."oct" ("format") enum16{"hex", "dec", "oct", "bin"}."bin" ("format")] -> w1644
                  frame "m002B", Default {
                  }
                  frame "m002A" {
                  }
                  frame "m0029" {
                  }
                  frame "m0028" {
                  }
                }
                n664 = call "sub-Get menu shortkey str.vi"("menu desc"=w1640) -> ("short key str"=w1637:string, "menu desc split"=w1639:string)  [unwired: 9 in]
                n665 = Concatenate Strings(w1639, "(%s)" ("字符串"), w1637) -> (w1636:string)
                n666 = invoke class="VI" method="Ctrl Val.Set"(reference=w1651, "Control Name"="format" ("控件名"), "Value"=w1644) -> (reference out=w1647:refnum<vi>)  [unwired: 2 in, 4 out]
                n667 = for {
                  shift-right: [w1670] -> w1650
                  shift-left: w1642 -> [w1671]
                  tunnel: string[] ["m002B", "m002A", "m0029", "m0028"] -> [w1669] mode=indexing
                  tunnel: w1657 -> [w1668]
                  tunnel: w1656 -> [w1667]
                  tunnel: w1655 -> [w1666]
                  tunnel: w1654 -> [w1665]
                  n668 = case shown="\"m0028\"" w1669 {
                    selector: w1669 -> [_ w1674 w1678 w1682 w1686]
                    tunnel: w1671 -> [w1672 w1676 w1680 w1684 w1688]
                    tunnel: [w1672 w1675 w1679 w1683 w1687] -> w1670
                    tunnel: w1668 -> [_ w1673 _ _ _]
                    tunnel: w1667 -> [_ _ w1677 _ _]
                    tunnel: w1666 -> [_ _ _ w1681 _]
                    tunnel: w1665 -> [_ _ _ _ w1685]
                    frame "", Default {
                    }
                    frame "m002B" {
                      n669 = Set Menu Item Info(6:w1673, 7:w1674, 11:w1676) -> (3:w1675:refnum<k9>)  [unwired: 4 in, 1 out]
                    }
                    frame "m002A" {
                      n670 = Set Menu Item Info(6:w1677, 7:w1678, 11:w1680) -> (3:w1679:refnum<k9>)  [unwired: 4 in, 1 out]
                    }
                    frame "m0029" {
                      n671 = Set Menu Item Info(6:w1681, 7:w1682, 11:w1684) -> (3:w1683:refnum<k9>)  [unwired: 4 in, 1 out]
                    }
                    frame "m0028" {
                      n672 = Set Menu Item Info(6:w1685, 7:w1686, 11:w1688) -> (3:w1687:refnum<k9>)  [unwired: 4 in, 1 out]
                    }
                  }
                }
                n673 = Format Into String(format string=w1636, w1644) -> (resulting string=w1648:string)  [unwired: 2 in, 1 out]
                n674 = invoke class="VI" method="Ctrl Val.Set"(reference=w1647, "Control Name"="ForceUpt" ("控件名"), "Value"=TRUE) -> ()  [unwired: 2 in, 5 out]
                n675 = Bundle By Name(cluster=w1661, "format"=w1644) -> (w1660:T2)
                n676 = Set Menu Item Info(7:"m001D" ("项标识符"), 10:w1648, 11:w1650) -> ()  [unwired: 4 in, 2 out]
              }
              frame "m002C" {
                n677 = Get Menu Item Info(7:w1722, 11:w1723) -> (3:w1725:refnum<k9>, 4:w1724:bool)  [unwired: 1 in, 5 out]
                n678 = Not(x=w1724) -> (.not. x?=w1712:bool)
                n679 = Set Menu Item Info(6:w1712, 7:w1722, 11:w1725) -> ()  [unwired: 4 in, 2 out]
                n680 = invoke class="VI" method="Ctrl Val.Set"(reference=w1721, "Control Name"="Rrate1" ("控件名"), "Value"=w1712) -> ()  [unwired: 2 in, 5 out]
                n681 = property on="Rrate1" class="DigNum (严格)"() -> ("Value"=w1711:dbl)  [unwired: 2 in, 2 out]
                n682 = Select(t=T4."Enabled" ("禁用"), s=w1712, f=T4."Disabled and Grayed Out" ("禁用")) -> (s? t:f=w1713:T4)
                n683 = Bundle By Name(cluster=w1718, "rateR1"=w1712) -> (w1719:T2)
                n684 = Select(t=w1711, s=w1712, f=0.0) -> (s? t:f=w1709:dbl)
                n685 = property on="Rrate1" class="DigNum (严格)"("DisabledEnum"=w1713, "Value"=w1709) -> ()  [unwired: 2 in, 2 out]
              }
              frame "m002D" {
                n686 = Get Menu Item Info(7:w1746, 11:w1747) -> (3:w1749:refnum<k9>, 4:w1748:bool)  [unwired: 1 in, 5 out]
                n687 = Not(x=w1748) -> (.not. x?=w1731:bool)
                n688 = Set Menu Item Info(6:w1731, 7:w1746, 11:w1749) -> ()  [unwired: 4 in, 2 out]
                n689 = Unbundle By Name(w1730) -> ("type"=w1734:u16)
                n690 = Equal?(x=u16 4, y=w1734) -> (x = y?=w1732:bool)
                n691 = property on="Rrate2" class="DigNum (严格)"() -> ("Value"=w1737:dbl)  [unwired: 2 in, 2 out]
                n692 = And(x=w1732, y=w1731) -> (x .and. y?=w1729:bool)
                n693 = invoke class="VI" method="Ctrl Val.Set"(reference=w1745, "Control Name"="Rrate2" ("控件名"), "Value"=w1729) -> ()  [unwired: 2 in, 5 out]
                n694 = Bundle By Name(cluster=w1730, "rateR2"=w1731) -> (w1743:T2)
                n695 = Select(t=w1737, s=w1729, f=0.0) -> (s? t:f=w1735:dbl)
                n696 = Select(t=T4."Enabled" ("禁用"), s=w1729, f=T4."Disabled and Grayed Out" ("禁用")) -> (s? t:f=w1738:T4)
                n697 = property on="Rrate2" class="DigNum (严格)"("DisabledEnum"=w1738, "Value"=w1735) -> ()  [unwired: 2 in, 2 out]
              }
              frame "m002E" {
                n698 = Get Menu Item Info(7:w1766, 11:w1767) -> (3:w1769:refnum<k9>, 4:w1768:bool)  [unwired: 1 in, 5 out]
                n699 = Not(x=w1768) -> (.not. x?=w1756:bool)
                n700 = Set Menu Item Info(6:w1756, 7:w1766, 11:w1769) -> ()  [unwired: 4 in, 2 out]
                n701 = invoke class="VI" method="Ctrl Val.Set"(reference=w1765, "Control Name"="Trate1" ("控件名"), "Value"=w1756) -> ()  [unwired: 2 in, 5 out]
                n702 = property on="Trate1" class="DigNum (严格)"() -> ("Value"=w1755:dbl)  [unwired: 2 in, 2 out]
                n703 = Select(t=T4."Enabled" ("禁用"), s=w1756, f=T4."Disabled and Grayed Out" ("禁用")) -> (s? t:f=w1757:T4)
                n704 = Bundle By Name(cluster=w1762, "rateT1"=w1756) -> (w1763:T2)
                n705 = Select(t=w1755, s=w1756, f=0.0) -> (s? t:f=w1753:dbl)
                n706 = property on="Trate1" class="DigNum (严格)"("DisabledEnum"=w1757, "Value"=w1753) -> ()  [unwired: 2 in, 2 out]
              }
              frame "m002F" {
                n707 = Get Menu Item Info(7:w1790, 11:w1791) -> (3:w1793:refnum<k9>, 4:w1792:bool)  [unwired: 1 in, 5 out]
                n708 = Not(x=w1792) -> (.not. x?=w1775:bool)
                n709 = Set Menu Item Info(6:w1775, 7:w1790, 11:w1793) -> ()  [unwired: 4 in, 2 out]
                n710 = Unbundle By Name(w1774) -> ("type"=w1778:u16)
                n711 = Equal?(x=u16 4, y=w1778) -> (x = y?=w1776:bool)
                n712 = property on="Trate2" class="DigNum (严格)"() -> ("Value"=w1781:dbl)  [unwired: 2 in, 2 out]
                n713 = And(x=w1776, y=w1775) -> (x .and. y?=w1773:bool)
                n714 = invoke class="VI" method="Ctrl Val.Set"(reference=w1789, "Control Name"="Trate2" ("控件名"), "Value"=w1773) -> ()  [unwired: 2 in, 5 out]
                n715 = Bundle By Name(cluster=w1774, "rateT2"=w1775) -> (w1787:T2)
                n716 = Select(t=w1781, s=w1773, f=0.0) -> (s? t:f=w1779:dbl)
                n717 = Select(t=T4."Enabled" ("禁用"), s=w1773, f=T4."Disabled and Grayed Out" ("禁用")) -> (s? t:f=w1782:T4)
                n718 = property on="Trate2" class="DigNum (严格)"("DisabledEnum"=w1782, "Value"=w1779) -> ()  [unwired: 2 in, 2 out]
              }
              frame "m0022" {
                n719 = Concatenate Strings("USB-CAN Tool V", w1797) -> (w1798:string)
                n720 = call "USB_CAN_ABOUT_DLG.vi"("Verinfo"=w1798) -> ()  [unwired: 11 in]
              }
              frame "m0032" {
                n721 = global read "sub-Language global.vi" "languages"() -> (w1809:T6)
                n722 = local read "selected"() -> (w1808:i32)
                n723 = call "Global_Application Path.vi"() -> ("程序路径"=w1811:path)  [unwired: 1 in]
                n724 = Index Array(array=w1809, index=w1808) -> (element=w1807:T8)
                n725 = Unbundle By Name(w1807) -> ("help dir"=w1806:string)
                n726 = Build Path(base path=w1811, name or relative path=w1806) -> (appended path=w1810:path)
                n727 = call "Launch a File with its Default Application.vi"("File Path"=w1810) -> ()  [unwired: 10 in, 1 out]
              }
              frame "m0033", "m0034", "m0035" {
                n728 = Scan From String(input string=w1828, initial scan location=u32 4 ("初始扫描位置"), default 1=0 ("默认值 1")) -> (output 1=w1820:i32)  [unwired: 2 in, 3 out]
                n729 = Subtract(x=w1820, y=3) -> (x-y=w1818:i32)
                n730 = Index Array(array=string[] ["3.USB-CAN Tool使用说明.pdf", "4.波特率侦测工具使用说明书.pdf", "5.中继、透明传输功能与中继软件使用说明(仅至尊版支持).pdf"], index=w1818) -> (element=w1823:string)
                n731 = Concatenate Strings("help" ("名称或相对路径"), "\\" ("字符串"), w1823) -> (w1821:string)
                n732 = call "Global_Application Path.vi"() -> ("程序路径"=w1830:path)  [unwired: 1 in]
                n733 = Build Path(base path=w1830, name or relative path=w1821) -> (appended path=w1829:path)
                n734 = call "Launch a File with its Default Application.vi"("File Path"=w1829) -> ()  [unwired: 10 in, 1 out]
              }
            }
          }
          event User Event {
            n735 = event-data() -> ("openCan"=w1840:bool)  [unwired: 1 in]
            n736 = call "FindUSBDevice.vi"("DevSNin"="") -> ("DevSN"=w1844:string, "DevNum"=w1846:i32)  [unwired: 6 in, 3 out]
            n737 = case shown="0.." w1846 {
              selector: w1846 -> [_ w1883]
              tunnel: [_ w1902] -> w1857
              tunnel: [w1868 w1901] -> w1855
              tunnel: w1854 -> [w1873 w1900]
              tunnel: [w1873 w1899] -> w1853
              tunnel: w1852 -> [w1872 w1898]
              tunnel: w1851 -> [_ w1897]
              tunnel: [w1872 w1885] -> w1850
              tunnel: [w1874 w1890] -> w1849
              tunnel: w1848 -> [_ w1889]
              tunnel: w1845 -> [w1874 _]
              tunnel: w1844 -> [_ w1887]
              tunnel: w1840 -> [_ w1882]
              tunnel: [5 ("time(s)") w1876] -> w1843
              tunnel: [_ w1875] -> w1839
              frame -1, Default {
                n738 = local write "brgsta"(u16 0 ("brgsta")) -> ()
                n739 = call "sub-Language-get str-const.vi"("sid"=u32 271) -> ("str"=w1868:string)
              }
              frame 0.. {
                n740 = Not(x=w1882) -> (.not. x?=w1881:bool)
                n741 = Unbundle By Name(w1897) -> ("autoconn"=w1879:bool, "RcvLen"=w1886:i16, "RcvE1"=w1896:bool, "RcvE2"=w1893:bool, "type"=w1895:u16)
                n742 = And(x=w1879, y=w1881) -> (x .and. y?=w1880:bool)
                n743 = call "PreOpenDevice.vi"("aotuConn?"=w1880, "Index"=w1883, "type"=w1889, "param"=w1898) -> ("Channels"=w1888:u32[], "DevIndex"=w1890:u32, "param out"=w1885:T5[])  [unwired: 5 in]
                n744 = Equal?(x=w1895, y=u16 4) -> (x = y?=w1891:bool)
                n745 = And(x=w1893, y=w1891) -> (x .and. y?=w1892:bool)
                n746 = call "OpenDevice.vi"("RcvLen"=w1886, "Enable2"=w1892, "DevIndex"=w1890, "Enable1"=w1896, "param"=w1885, "Channels"=w1888, "type"=w1889) -> ("bridge type"=w1877:T9, "Error info"=w1878:string, "open"=w1902:bool)  [unwired: 1 in, 1 out]
                n747 = case shown="假" w1902 {
                  tunnel: [w1909 w1911] -> w1901
                  tunnel: w1900 -> [w1910 w1928]
                  tunnel: [w1910 w1927] -> w1899
                  tunnel: w1889 -> [_ w1923]
                  tunnel: w1887 -> [_ w1925]
                  tunnel: w1883 -> [_ w1922]
                  tunnel: w1878 -> [w1904 _]
                  tunnel: w1877 -> [_ w1919]
                  tunnel: [5 ("time(s)") w1917] -> w1876
                  tunnel: [w1903 _] -> w1875
                  frame False {
                    n748 = Empty String/Path?(string/path=w1904) -> (empty?=w1903:bool)
                    n749 = call "sub-Language-get str-const.vi"("sid"=u32 274) -> ("str"=w1905:string)
                    n750 = Concatenate Strings(w1905, w1904) -> (w1909:string)
                    n751 = local write "brgsta"(u16 0 ("brgsta")) -> ()
                  }
                  frame True {
                    w1926 = " - " ("字符串")
                    n752 = call "ReadBoardInfo.vi"("DeviceInd"=w1922, "DeviceType"=w1923) -> ("VCI_BOARD_INFO"=w1921:T7)  [unwired: 8 in, 1 out]
                    n753 = Greater Than 0?(x=w1919) -> (x > 0?=w1918:bool)
                    n754 = Unbundle By Name(w1921) -> ("str_hw_Type"=w1920:string)
                    n755 = Select(t=u32 272 ("sid"), s=w1918, f=u32 273 ("sid")) -> (s? t:f=w1912:u32)
                    n756 = Concatenate Strings(w1928, w1926, w1920, w1926, "SN:" ("字符串"), w1925) -> (w1927:string)
                    n757 = Select(t=20 ("time(s)"), s=w1918, f=5 ("time(s)")) -> (s? t:f=w1917:i32)
                    n758 = call "sub-Language-get str-const.vi"("sid"=w1912) -> ("str"=w1911:string)
                    "brgsta" <- w1919
                  }
                }
                n759 = call "_USB_CAN_PARAM_RW_.vi"("write"=TRUE, "param"=w1885) -> ()  [unwired: 9 in, 1 out]
              }
            }
            "DevIndex" <- w1849
            n760 = Not(x=w1839) -> (.not. x?=w1837:bool)
            n761 = And(x=w1837, y=w1840) -> (x .and. y?=w1838:bool)
            n762 = global write "_USB_CAN_GLOBAL_.vi" "open"(w1857) -> ()
            n763 = call "sub-Language-get str-const.vi"("sid"=u32 256) -> ("str"=w1841:string)
            n764 = property class="VI"("Front Panel.Title"=w1853) -> ()  [unwired: 2 in, 2 out]
            n765 = case shown="真" w1838 {
              tunnel: w1841 -> [_ w1931]
              tunnel: w1855 -> [_ w1930]
              tunnel: w1843 -> [_ w1929]
              frame False {
              }
              frame True {
                n766 = call "TimeLmtDialog.vi"("time(s)"=w1929, "Infoin"=w1930, "title"=w1931) -> ()  [unwired: 9 in]
              }
            }
          }
          event Panel Close? {
            n767 = event-data() -> ()  [unwired: 1 in, 1 out]
            n768 = event-data("Discard?"=TRUE ("放弃？")) -> ()  [unwired: 1 in, 1 out]
          }
          event "sendfile": Value Change {
            n769 = event-data() -> ()  [unwired: 1 in, 1 out]
            n770 = case shown="假" w1952 {
              tunnel: w1954 -> [_ w1988]
              tunnel: w1949 -> [_ w1970]
              frame False {
                n771 = call "sub-Language-get str-const.vi"("sid"=u32 256) -> ("str"=w1968:string)
                n772 = call "sub-Language-get str-const.vi"("sid"=u32 270) -> ("str"=w1966:string)
                n773 = call "TimeLmtDialog.vi"("Infoin"=w1966, "title"=w1968) -> ()  [unwired: 10 in]
              }
              frame True {
                n774 = invoke class="VI" method="Ctrl Val.Set"(reference=w1988, "Control Name"="sendfile" ("控件名"), "Value"=TRUE) -> (reference out=w1984:refnum<vi>, error out=w1978:errorcluster)  [unwired: 2 in, 3 out]
                n775 = local read "SendCnt"() -> (w1981:i32)
                n776 = invoke class="VI" method="Ctrl Val.Set"(reference=w1984, error in=w1978, "Control Name"="FrameCnt" ("控件名"), "Value"=w1981) -> (reference out=w1980:refnum<vi>, error out=w1979:errorcluster)  [unwired: 1 in, 3 out]
                n777 = local read "sendcycle"() -> (w1974:i32)
                n778 = invoke class="VI" method="Ctrl Val.Set"(reference=w1980, error in=w1979, "Control Name"="Cycle" ("控件名"), "Value"=w1974) -> (reference out=w1976:refnum<vi>, error out=w1977:errorcluster)  [unwired: 1 in, 3 out]
                n779 = invoke class="VI" method="Ctrl Val.Set"(reference=w1976, error in=w1977, "Control Name"="Enable" ("控件名"), "Value"=TRUE) -> (reference out=w1973:refnum<vi>, error out=w1972:errorcluster)  [unwired: 1 in, 3 out]
                n780 = invoke class="VI" method="Ctrl Val.Set"(reference=w1973, error in=w1972, "Control Name"="channel" ("控件名"), "Value"=w1970) -> ()  [unwired: 1 in, 5 out]
              }
            }
          }
          event "savefile": Value Change {
            n781 = event-data() -> ()  [unwired: 1 in, 1 out]
            n782 = invoke class="VI" method="Ctrl Val.Set"(reference=w1996, "Control Name"="save" ("控件名"), "Value"="savefile") -> (reference out=w1991:refnum<vi>, error out=w1990:errorcluster)  [unwired: 2 in, 3 out]
            n783 = invoke class="VI" method="Ctrl Val.Set"(reference=w1991, error in=w1990, "Control Name"="sPth_Sel" ("控件名"), "Value"="savefile") -> ()  [unwired: 1 in, 5 out]
            n784 = disable-structure shown="禁用" {
              disable-tunnel: w1993 -> [w2015 _]
              disable-tunnel: "savefile" -> [w2014 _]
              frame Disabled {
                n785 = Set Menu Item Info(6:w2014, 7:"m4_2" ("控件名"), 11:w2015) -> ()  [unwired: 4 in, 2 out]
              }
              frame Enabled {
              }
            }
            n786 = Bundle By Name(cluster=w1995, "save"="savefile") -> (w1994:T2)
            n787 = property on="path" class="Path"("Value"=path "" ("path")) -> ()  [unwired: 2 in, 2 out]
          }
          event "clear": Value Change {
            n788 = event-data() -> ()  [unwired: 1 in, 1 out]
            n789 = stacked-sequence {
              tunnel: w2024 -> [w2040]
              tunnel: [w2038] -> w2019
              frame #0 {
                n790 = invoke class="VI" method="Ctrl Val.Set"(reference=w2040, "Control Name"="clear" ("控件名"), "Value"=TRUE) -> (reference out=w2038:refnum<vi>)  [unwired: 2 in, 4 out]
                n791 = Wait (ms)(milliseconds to wait=u32 100 ("等待时间（毫秒）")) -> ()  [unwired: 1 out]
              }
            }
            n792 = invoke class="VI" method="Ctrl Val.Set"(reference=w2019, "Control Name"="listcount" ("控件名"), "Value"=u32 0) -> ()  [unwired: 2 in, 5 out]
          }
          event "reciveEnable": Value Change {
            n793 = event-data() -> ("NewVal"=w2042:bool)  [unwired: 1 in]
            n794 = invoke class="VI" method="Ctrl Val.Set"(reference=w2048, "Control Name"="Enable" ("控件名"), "Value"=w2042) -> ()  [unwired: 2 in, 5 out]
            n795 = global write "_USB_CAN_GLOBAL_.vi" "R-Enb"(w2042) -> ()
          }
          event "Send": Value Change {
            n796 = event-data() -> ()  [unwired: 1 in, 1 out]
            n797 = case shown="假" w2065 {
              tunnel: w2070 -> [_ w2086]
              tunnel: w2069 -> [_ w2085]
              tunnel: w2068 -> [_ w2084]
              tunnel: w2067 -> [_ w2083]
              tunnel: w2061 -> [_ w2082]
              frame False {
                n798 = call "sub-Language-get str-const.vi"("sid"=u32 256) -> ("str"=w2080:string)
                n799 = call "sub-Language-get str-const.vi"("sid"=u32 270) -> ("str"=w2078:string)
                n800 = call "TimeLmtDialog.vi"("Infoin"=w2078, "title"=w2080) -> ()  [unwired: 10 in]
              }
              frame True {
                w2088 = T4."Disabled and Grayed Out" ("禁用")
                n801 = property on="send stop" class="Bool (严格)"("DisabledEnum"=T4."Enabled" ("禁用")) -> ()  [unwired: 2 in, 2 out]
                n802 = property on="Send" class="Bool"("DisabledEnum"=w2088) -> ()  [unwired: 2 in, 2 out]
                n803 = property on="data" class="Str"("DisabledEnum"=w2088) -> ()  [unwired: 2 in, 2 out]
                n804 = property on="ID Inc" class="Bool (严格)"("DisabledEnum"=w2088) -> ()  [unwired: 2 in, 2 out]
                n805 = property on="sendcycle" class="DigNum (严格)"("DisabledEnum"=w2088) -> ()  [unwired: 2 in, 2 out]
                n806 = property on="Data Inc" class="Bool (严格)"("DisabledEnum"=w2088) -> ()  [unwired: 2 in, 2 out]
                n807 = property on="SendCnt" class="DigNum (严格)"("DisabledEnum"=w2088) -> ()  [unwired: 2 in, 2 out]
                n808 = for {
                  N: 10 -> [_]
                  tunnel: w2086 -> [w2094]
                  tunnel: w2085 -> [w2093]
                  tunnel: w2084 -> [w2092]
                  tunnel: w2083 -> [w2091]
                  tunnel: w2082 -> [w2090]
                  i -> [w2095]
                  n809 = case shown="9" w2095 {
                    tunnel: w2094 -> [_ w2098 w2101 w2104 w2107 w2110 w2113 w2117 w2121 w2124 w2127]
                    tunnel: w2093 -> [_ w2096 _ _ _ _ _ _ _ _ _]
                    tunnel: w2092 -> [_ _ w2099 _ _ _ _ _ _ _ _]
                    tunnel: w2091 -> [_ _ _ _ _ _ w2111 _ _ _ _]
                    tunnel: w2090 -> [_ _ _ _ _ _ _ _ _ _ w2125]
                    frame -1, Default {
                    }
                    frame 0 {
                      n810 = invoke class="VI" method="Ctrl Val.Set"(reference=w2098, "Control Name"="data" ("控件名"), "Value"=w2096) -> ()  [unwired: 2 in, 5 out]
                    }
                    frame 1 {
                      n811 = invoke class="VI" method="Ctrl Val.Set"(reference=w2101, "Control Name"="FrameCnt" ("控件名"), "Value"=w2099) -> ()  [unwired: 2 in, 5 out]
                    }
                    frame 2 {
                      n812 = invoke class="VI" method="Ctrl Val.Set"(reference=w2104, "Control Name"="Cycle" ("控件名"), "Value"="sendcycle") -> ()  [unwired: 2 in, 5 out]
                    }
                    frame 3 {
                      n813 = invoke class="VI" method="Ctrl Val.Set"(reference=w2107, "Control Name"="ID Inc" ("控件名"), "Value"="ID Inc") -> ()  [unwired: 2 in, 5 out]
                    }
                    frame 4 {
                      n814 = invoke class="VI" method="Ctrl Val.Set"(reference=w2110, "Control Name"="Data Inc" ("控件名"), "Value"="Data Inc") -> ()  [unwired: 2 in, 5 out]
                    }
                    frame 5 {
                      n815 = invoke class="VI" method="Ctrl Val.Set"(reference=w2113, "Control Name"="ID" ("控件名"), "Value"=w2111) -> ()  [unwired: 2 in, 5 out]
                    }
                    frame 6 {
                      n816 = local read "Frame Format"() -> (w2115:u16)
                      n817 = Not Equal To 0?(x=w2115) -> (x != 0?=w2114:bool)
                      n818 = invoke class="VI" method="Ctrl Val.Set"(reference=w2117, "Control Name"="ExtFrame" ("控件名"), "Value"=w2114) -> ()  [unwired: 2 in, 5 out]
                    }
                    frame 7 {
                      n819 = local read "Frame Type"() -> (w2118:u16)
                      n820 = Not Equal To 0?(x=w2118) -> (x != 0?=w2119:bool)
                      n821 = invoke class="VI" method="Ctrl Val.Set"(reference=w2121, "Control Name"="remote" ("控件名"), "Value"=w2119) -> ()  [unwired: 2 in, 5 out]
                    }
                    frame 8 {
                      n822 = invoke class="VI" method="Ctrl Val.Set"(reference=w2124, "Control Name"="Enable" ("控件名"), "Value"=TRUE) -> ()  [unwired: 2 in, 5 out]
                    }
                    frame 9 {
                      n823 = invoke class="VI" method="Ctrl Val.Set"(reference=w2127, "Control Name"="channel" ("控件名"), "Value"=w2125) -> ()  [unwired: 2 in, 5 out]
                    }
                  }
                }
              }
            }
          }
          event "send stop": Value Change {
            w2130 = FALSE
            w2138 = T4."Enabled" ("禁用")
            n824 = event-data() -> ()  [unwired: 1 in, 1 out]
            n825 = Not(x=w2130) -> (.not. x?=w2129:bool)
            n826 = invoke class="VI" method="Ctrl Val.Set"(reference=w2134, "Control Name"="Enable" ("控件名"), "Value"=w2130) -> ()  [unwired: 2 in, 5 out]
            n827 = global write "_USB_CAN_GLOBAL_.vi" "S-Cancel"(w2129) -> ()
            n828 = property on="send stop" class="Bool (严格)"("DisabledEnum"=T4."Disabled and Grayed Out" ("禁用")) -> ()  [unwired: 2 in, 2 out]
            n829 = property on="Send" class="Bool"("DisabledEnum"=w2138) -> ()  [unwired: 2 in, 2 out]
            n830 = property on="data" class="Str"("DisabledEnum"=w2138) -> ()  [unwired: 2 in, 2 out]
            n831 = property on="ID Inc" class="Bool (严格)"("DisabledEnum"=w2138) -> ()  [unwired: 2 in, 2 out]
            n832 = property on="sendcycle" class="DigNum (严格)"("DisabledEnum"=w2138) -> ()  [unwired: 2 in, 2 out]
            n833 = property on="Data Inc" class="Bool (严格)"("DisabledEnum"=w2138) -> ()  [unwired: 2 in, 2 out]
            n834 = property on="SendCnt" class="DigNum (严格)"("DisabledEnum"=w2138) -> ()  [unwired: 2 in, 2 out]
            n835 = local write "send stop"(FALSE ("send stop")) -> ()
          }
          event "ID Filter Set": Value Change {
            n836 = event-data() -> ()  [unwired: 1 in, 1 out]
            n837 = call "str_to_u32_arr.vi"("string"="ID Filter Str") -> ("array"=w2151:u32[])
            n838 = Select(t=w2151, s=w2163, f=w2166) -> (s? t:f=w2161:u32[])
            n839 = invoke class="VI" method="Ctrl Val.Set"(reference=w2156, "Control Name"="UseFilter" ("控件名"), "Value"=TRUE) -> (reference out=w2157:refnum<vi>)  [unwired: 2 in, 4 out]
            n840 = invoke class="VI" method="Ctrl Val.Set"(reference=w2157, "Control Name"="Filter" ("控件名"), "Value"=w2161) -> ()  [unwired: 2 in, 5 out]
          }
          event "ID Filter": Value Change {
            n841 = event-data() -> ("NewVal"=w2188:enum32{"enable", "disable"})  [unwired: 1 in]
            n842 = Equal?(x=w2188, y=enum32{"enable", "disable"}."enable") -> (x = y?=w2178:bool)
            n843 = Select(t=T4."Enabled" ("禁用"), s=w2178, f=T4."Disabled and Grayed Out" ("禁用")) -> (s? t:f=w2184:T4)
            n844 = property on="ID Filter Str" class="Str"("DisabledEnum"=w2184) -> ()  [unwired: 2 in, 2 out]
            n845 = property on="ID Filter Set" class="Bool"("DisabledEnum"=w2184) -> ()  [unwired: 2 in, 2 out]
            n846 = case shown="假" w2178 {
              selector: w2178 -> [w2197 _]
              tunnel: w2181 -> [w2201 _]
              tunnel: w2180 -> [w2198 _]
              frame False {
                n847 = invoke class="VI" method="Ctrl Val.Set"(reference=w2201, "Control Name"="UseFilter" ("控件名"), "Value"=w2197) -> (reference out=w2199:refnum<vi>)  [unwired: 2 in, 4 out]
                n848 = invoke class="VI" method="Ctrl Val.Set"(reference=w2199, "Control Name"="Filter" ("控件名"), "Value"=w2198) -> ()  [unwired: 2 in, 5 out]
              }
              frame True {
              }
            }
          }
          event "data": Value Change {
            n849 = event-data() -> ("NewVal"=w2208:string)  [unwired: 1 in]
            n850 = call "str_to_u32_arr.vi"("string"=w2208) -> ("array"=w2207:u32[])
            n851 = To Unsigned Byte Integer(number=w2207) -> (unsigned 8bit integer=w2206:u8[])
          }
          event "SendCnt": Value Change {
            n852 = event-data() -> ("NewVal"=w2227:i32)  [unwired: 1 in]
          }
          event "CAN Channel": Value Change {
            n853 = event-data() -> ("NewVal"=w2243:u16)  [unwired: 1 in]
          }
          event "Frame ID": Value Change {
            n854 = event-data() -> ("NewVal"=w2260:string)  [unwired: 1 in]
            n855 = call "FormatIDString.vi"("ID String"=w2260) -> ("ID"=w2259:u32)
          }
          event "Frame Type": Value Change {
            n856 = event-data() -> ("NewVal"=w2276:u16)  [unwired: 1 in]
          }
          event "Frame Format": Value Change {
            n857 = event-data() -> ("NewVal"=w2292:u16)  [unwired: 1 in]
          }
          event "list": Mouse Down {
            n858 = event-data() -> ("CtlRef"=w2315:refnum<vi>, "Coords"=w2314:T10)  [unwired: 1 in]
            n859 = invoke class="MCListbox (严格)" method="Point To Row Column"(reference=w2315, "Point"=w2314) -> (reference out=w2313:refnum<vi>, "InBounds"=w2304:bool, "CellPosition"=w2310:T11)  [unwired: 5 in, 4 out]
            n860 = Unbundle By Name(w2310) -> ("Row"=w2308:i32)
            n861 = property class="MCListbox (严格)"(reference=w2313) -> (reference out=w2302:refnum<vi>, "ItemNames"=w2312:string[][])  [unwired: 1 in, 1 out]
            n862 = Array Size(array=w2312) -> (size(s)=w2311:i32[])
            n863 = Index Array(array=w2311) -> (element=w2309:i32)  [unwired: 1 in]
            n864 = Greater Than 0?(x=w2309) -> (x > 0?=w2307:bool)
            n865 = Greater?(x=w2309, y=w2308) -> (0:w2306:bool)
            n866 = And(x=w2307, y=w2306) -> (x .and. y?=w2305:bool)
            n867 = And(x=w2305, y=w2304) -> (x .and. y?=w2303:bool)
            n868 = case shown="假" w2303 {
              tunnel: w2302 -> [w2333 _]
              frame False {
                n869 = property class="MCListbox (严格)"(reference=w2333, "Value"=-1 ("值")) -> ()  [unwired: 1 in, 2 out]
              }
              frame True {
              }
            }
          }
        }
      }
      frame "unRegistEvent" {
        n870 = local read "DevIndex"() -> (w2335:u32)
        n871 = stacked-sequence {
          tunnel: w2334 -> [w2361 w2371]
          tunnel: w2335 -> [w2360 w2370]
          frame #0 {
            n872 = Equal?(x=w2361, y=u16 4) -> (x = y?=w2365:bool)
            n873 = Select(t=2, s=w2365, f=1) -> (s? t:f=w2362:i32)
            n874 = for {
              N: w2362 -> [_]
              tunnel: w2361 -> [w2369]
              tunnel: w2360 -> [w2368]
              i -> [w2367]
              n875 = call "ResetCAN.vi"("CANInd"=w2367, "DeciceInd"=w2368, "DeviceType"=w2369) -> ()  [unwired: 7 in, 2 out]
            }
          }
          frame #1 {
            n876 = call "CloseDevice.vi"("DeviceInd"=w2370, "type"=w2371) -> ()  [unwired: 8 in, 2 out]
          }
        }
        n877 = Unregister For Events(event registration refnum=w2348) -> (error out=w2347:errorcluster)  [unwired: 1 in]
        n878 = Destroy User Event(user event=w2346, error in=w2347) -> (error out=w2344:errorcluster)
        n879 = call "_USB_CAN_PARAM_RW_.vi"("write"=TRUE, "param"=w2342) -> ()  [unwired: 9 in, 1 out]
        n880 = Destroy User Event(user event=w2343, error in=w2344) -> (error out=w2338:errorcluster)
        n881 = Destroy User Event(user event=w2337, error in=w2338) -> ()  [unwired: 1 out]
        n882 = property class="VI"(reference=w2351) -> (reference out=w2353:refnum<vi>, "Exec.State"=w2352:T12)  [unwired: 1 in, 1 out]
        n883 = property class="VI"(reference=w2358) -> (reference out=w2356:refnum<vi>, "Exec.State"=w2357:T12)  [unwired: 1 in, 1 out]
        n884 = case shown="\"Run top level\", \"Running\"" w2352 {
          tunnel: w2353 -> [w2372 w2377]
          tunnel: [w2372 w2376] -> w2354
          frame "Bad", Default {
          }
          frame "Run top level", "Running" {
            n885 = invoke class="VI" method="Ctrl Val.Set"(reference=w2377, "Control Name"="stop" ("控件名"), "Value"=TRUE) -> (reference out=w2376:refnum<vi>, error out=w2373:errorcluster)  [unwired: 2 in, 3 out]
            n886 = call "0.1秒"("error in (no error)"=w2373) -> ()  [unwired: 10 in, 1 out]
          }
        }
        n887 = case shown="\"Run top level\", \"Running\"" w2357 {
          tunnel: w2356 -> [w2378 w2383]
          tunnel: [w2378 w2382] -> w2355
          frame "Bad", Default {
          }
          frame "Run top level", "Running" {
            n888 = invoke class="VI" method="Ctrl Val.Set"(reference=w2383, "Control Name"="stop" ("控件名"), "Value"=TRUE) -> (reference out=w2382:refnum<vi>, error out=w2379:errorcluster)  [unwired: 2 in, 3 out]
            n889 = call "0.1秒"("error in (no error)"=w2379) -> ()  [unwired: 10 in, 1 out]
          }
        }
        n890 = Close Reference(reference=w2354) -> ()  [unwired: 1 in, 1 out]
        n891 = Close Reference(reference=w2355) -> (error out=w2345:errorcluster)  [unwired: 1 in]
        n892 = global write "_USB_CAN_GLOBAL_.vi" "R-Enable"(FALSE ("R-Enable")) -> ()
        n893 = global write "_USB_CAN_GLOBAL_.vi" "S-Enable"(FALSE ("R-Enable")) -> ()
      }
      frame "Release" {
        n894 = call "ReciveBuffer.vi"("销毁?"=TRUE) -> ()  [unwired: 1 out]
        n895 = call "MonitorBuffer.vi"("销毁?"=TRUE) -> ()  [unwired: 1 out]
        n896 = call "SendBuffer.vi"("销毁"=TRUE) -> ()  [unwired: 1 out]
        n897 = control-ref of="本VI"() -> (w2386:refnum<vi>)
        n898 = call "UI_Status.vi"("write?"=TRUE, "menu status in"=w2385, "VI ref"=w2386) -> ()  [unwired: 7 in, 2 out]
      }
      frame "Exit" {
      }
    }
  }
  n899 = control-ref of="本VI"() -> (w12:refnum<vi>)
  n900 = call "Exit.vi"("error in (no error)"=w13, "VI引用"=w12) -> ()  [unwired: 9 in, 1 out]
